vi "Autonomous Independent.vi"() -> ()   [LabVIEW 2017]
doc: "This VI is called when autonomous begins, and will automatically be terminated when autonomous ends. You can carry out timed or sensor driven robot movement independently without needing to return to the caller."
uses:
  Public/Documents/Cross The Road Electronics/Phoenix-LabVIEW/Motor Controller/Controls/CTRE_Phoenix_MotorControl_ControlMode.ctl
  <vilib>/Rock Robotics/WPI/Solenoid/WPI_SolenoidValue.ctl
  <vilib>/Rock Robotics/WPI/Utilities/WPI_GetSetVariantRefNum.vi
  <vilib>/Rock Robotics/Network Tables/NT Read String.vi
  <vilib>/Rock Robotics/Network Tables/NT Write Numeric Array.vi
  <vilib>/Rock Robotics/WPI/RobotDrive/WPI_RobotDriveArcadeDrive_Standard(NoSaturation).vi
  <vilib>/addons/control/pid/pid.llb/PID (DBL).vi
  <vilib>/Rock Robotics/WPI/Solenoid/WPI_SolenoidSetEnum.vi
  <vilib>/addons/control/pid/NI_PID_pid.lvlib
  <vilib>/Rock Robotics/WPI/ThirdParty/Sensors/ADIS16448 IMU/ADIS16448_IMU.lvlib
panel:
  out "Current Movement, for debugging":T1 {"Y Joystick Value" scale=1.0..-1.0; "X Joystick Value" scale=-1.0..1.0}
  in  "Array of robot movements":T2(array[cluster])=[{"X Joystick Value"=0.39393939393939403, "Y Joystick Value"=0.0, "Delay (sec)"=1.0, "Movement Name"="turn"}, {"X Joystick Value"=-0.3737373737373737, "Y Joystick Value"=0.0, "Delay (sec)"=1.0, "Movement Name"="turn back"}] {"Y Joystick Value" scale=1.0..-1.0; "X Joystick Value" scale=-1.0..1.0}
  # "Be sure to right-click and choose Data Operations>>Make Current Value default if you want to save the array values with the VI"
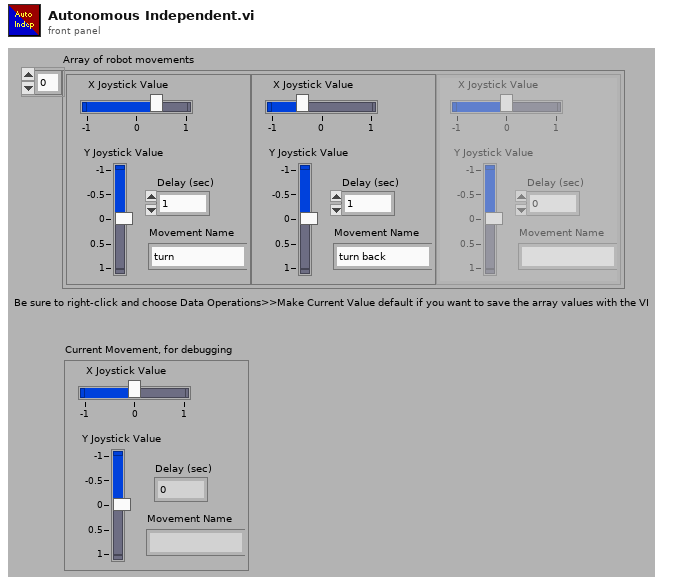
[diagram p1: front panel]
types:
  T1 = cluster{"X Joystick Value":dbl, "Y Joystick Value":dbl, "Delay (sec)":dbl, "Movement Name":string}
  T2 = cluster{"X Joystick Value":dbl, "Y Joystick Value":dbl, "Delay (sec)":dbl, "Movement Name":string}[]
  T3 = typedef "WPI_JoystickDevRef.ctl" = cluster{"Device":T4}
  T4 = typedef "WPI_JoystickDeviceEnum.ctl" = enum16{"USB 0", "USB 1", "USB 2", "USB 3", "USB 4", "USB 5"}
  T5 = typedef "ADIS16448_IMU.lvlib/ADI_IMU_ADIS16448_IMUDevRef.ctl" = cluster{"DevStatus":errorcluster, "Handle":i32, "SPI Bus":T6, "Device Found":bool, "Device Ready":bool, "Yaw Axis":enum16{"X", "Y", "Z"}, "AHRS Algorithm":enum16{"Complementary", "Madgwick"}, "Serial":u16, "Lot ID 2":u16, "Lot ID 1":u16, "Bytes Per Sample":u16, "Calibrate On Open?":bool}
  T6 = typedef "spi_bus.ctl" = enum16{"SPI On-Board, CS0", "SPI On-Board, CS1", "SPI On-Board, CS2", "SPI On-Board, CS3", "SPI MXP", "Invalid"}
  T7 = typedef "WPI_RobotDriveDevRef.ctl" = cluster{"DevStatus":errorcluster, "Motors[]":T8[], "Square Inputs":bool, "Max Output":dbl}
  T8 = typedef "WPI_MotorControlDeviceRef.ctl" = cluster{"DeviceStatus":errorcluster, "Type":T9, "PWM":cluster{"PWM Channel":T10, "DeadBand":T11}, "CAN":cluster{"Device Number":u8, "SetOutput VI Ref":variant, "GetOutput VI Ref":variant, "Enable VI Ref":variant, "Disable VI Ref":variant, "Data":variant}, "Invert":bool, "DIO PWM":cluster{"PWM \"Enable\" Channel":T10, "DIOChannel":T12, "PWM Rate":dbl}}
  T9 = typedef "WPI_MotorControlType.ctl" = enum16{"PWM", "CAN", "DIO PWM"}
  T10 = typedef "FPGA_DIOPWMChannel.ctl" = enum8{"PWM 0", "PWM 1", "PWM 2", "PWM 3", "PWM 4", "PWM 5", "PWM 6", "PWM 7", "PWM 8", "PWM 9", "PWM MXP 0", "PWM MXP 1", "PWM MXP 2", "PWM MXP 3", "PWM MXP 4", "PWM MXP 5", "PWM MXP 6", "PWM MXP 7", "PWM MXP 8", "PWM MXP 9", "Invalid"}
  T11 = typedef "WPI_PWMDeadband.ctl" = cluster{"Name":string, "maxPositivePwm":i32, "minPositivePwm":i32, "centerPwm":i32, "maxNegativePwm":i32, "minNegativePwm":i32, "angularRange":u16}
  T12 = typedef "FPGA_DIOChannel.ctl" = enum8{"DIO 0", "DIO 1", "DIO 2", "DIO 3", "DIO 4", "DIO 5", "DIO 6", "DIO 7", "DIO 8", "DIO 9", "DIO MXP 0", "DIO MXP 1", "DIO MXP 2", "DIO MXP 3", "DIO MXP 4", "DIO MXP 5", "DIO MXP 6", "DIO MXP 7", "DIO MXP 8", "DIO MXP 9", "DIO MXP 10", "DIO MXP 11", "DIO MXP 12", "DIO MXP 13", "DIO MXP 14", "DIO MXP 15", "SPI Port CS1", "SPI Port CS2", "SPI Port CS3", "SPI Port MISO", "SPI Port MOSI", "Invalid"}
  T13 = typedef "WPI_SolenoidDevRef.ctl" = cluster{"DevStatus":errorcluster, "Pneumatics Control Module":u8, "Forward Solenoid Channel":T14, "Reverse Solenoid Channel":T14}
  T14 = typedef "WPI_SolenoidChannel.ctl" = enum8{"Solenoid 0", "Solenoid 1", "Solenoid 2", "Solenoid 3", "Solenoid 4", "Solenoid 5", "Solenoid 6", "Solenoid 7", "Invalid"}
  T15 = cluster{"proportional gain (Kc)":dbl, "integral time (Ti, min)":dbl, "derivative time (Td, min)":dbl}
  T16 = typedef "WPI_SolenoidValue.ctl" = enum16{"Off", "On", "Forward", "Reverse"}
  T17 = cluster{"X Angle":dbl, "Y Angle":dbl, "Z Angle":dbl}
  T18 = typedef "CTRE_Phoenix_MotorControl_ControlMode.ctl" = u16
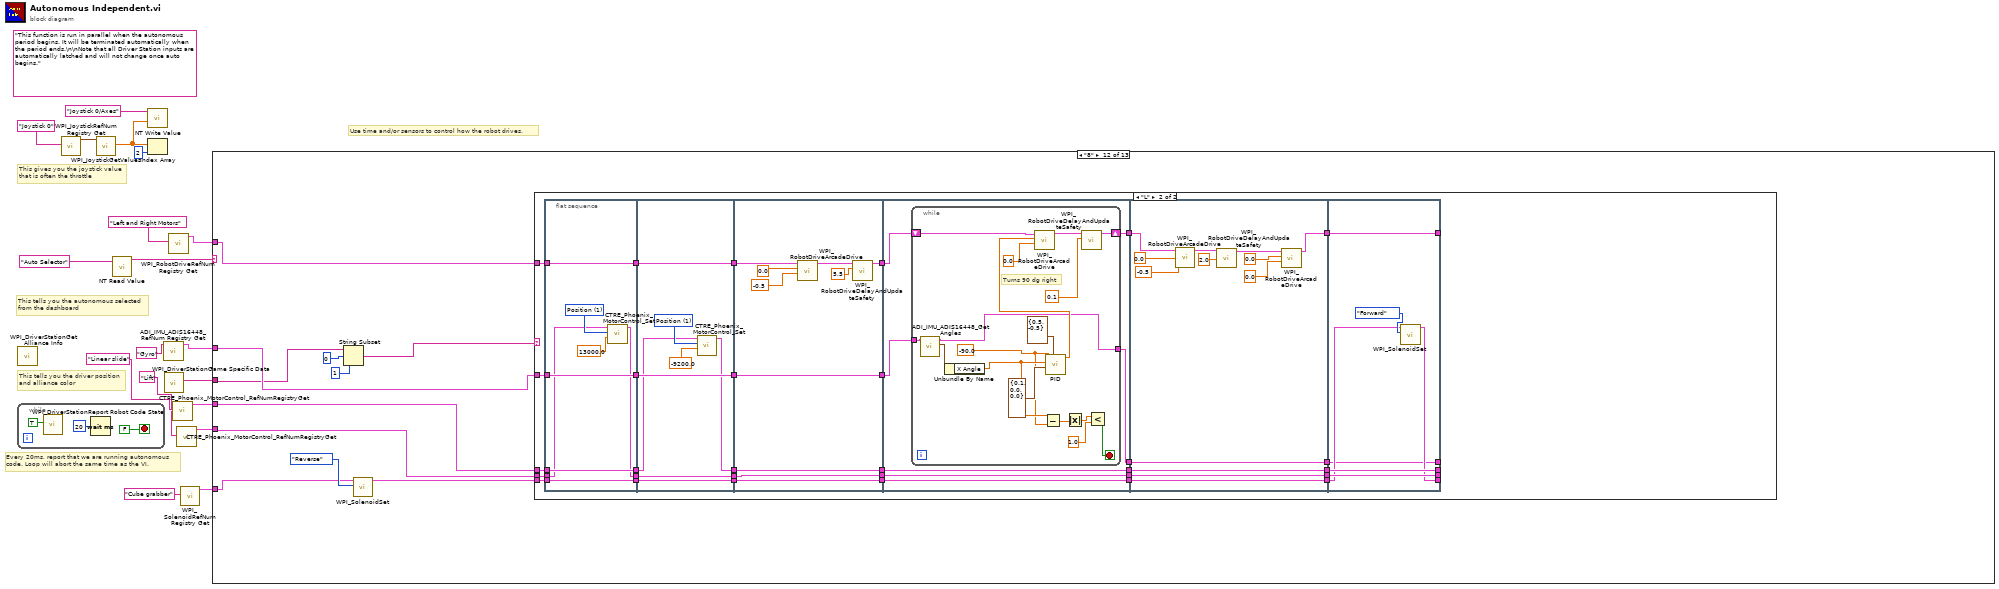
[diagram p0: block diagram]
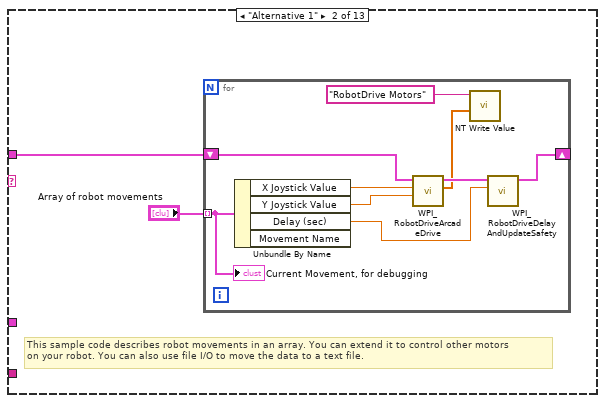
[diagram p3: hidden frame]
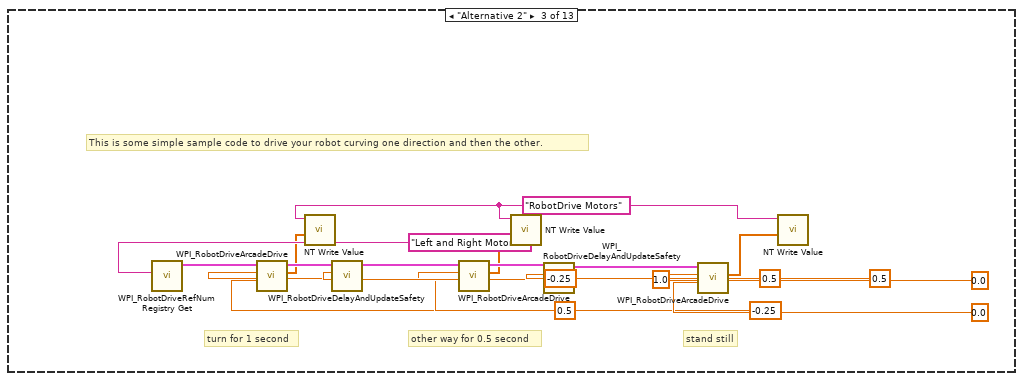
[diagram p4: hidden frame]
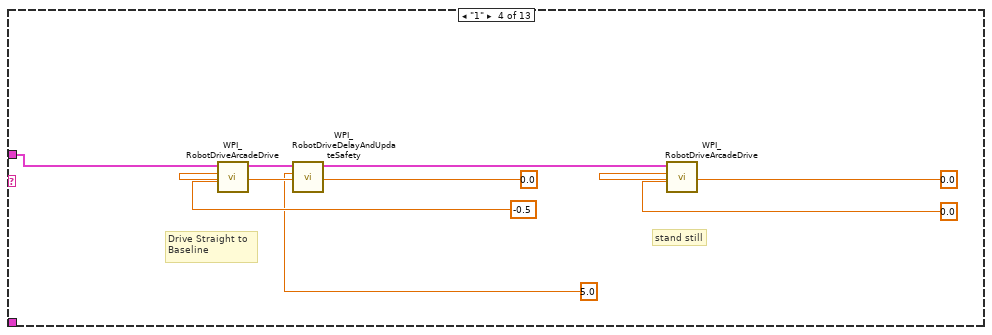
[diagram p5: hidden frame]
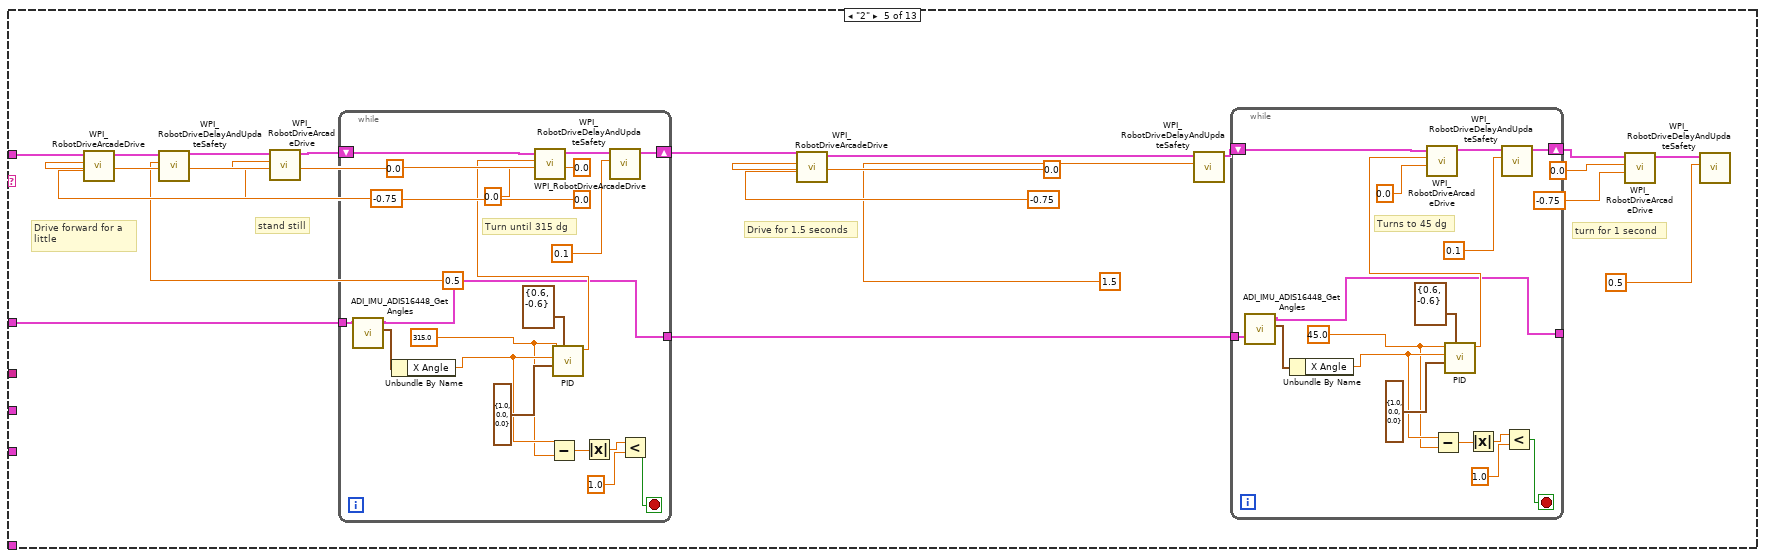
[diagram p6: hidden frame]
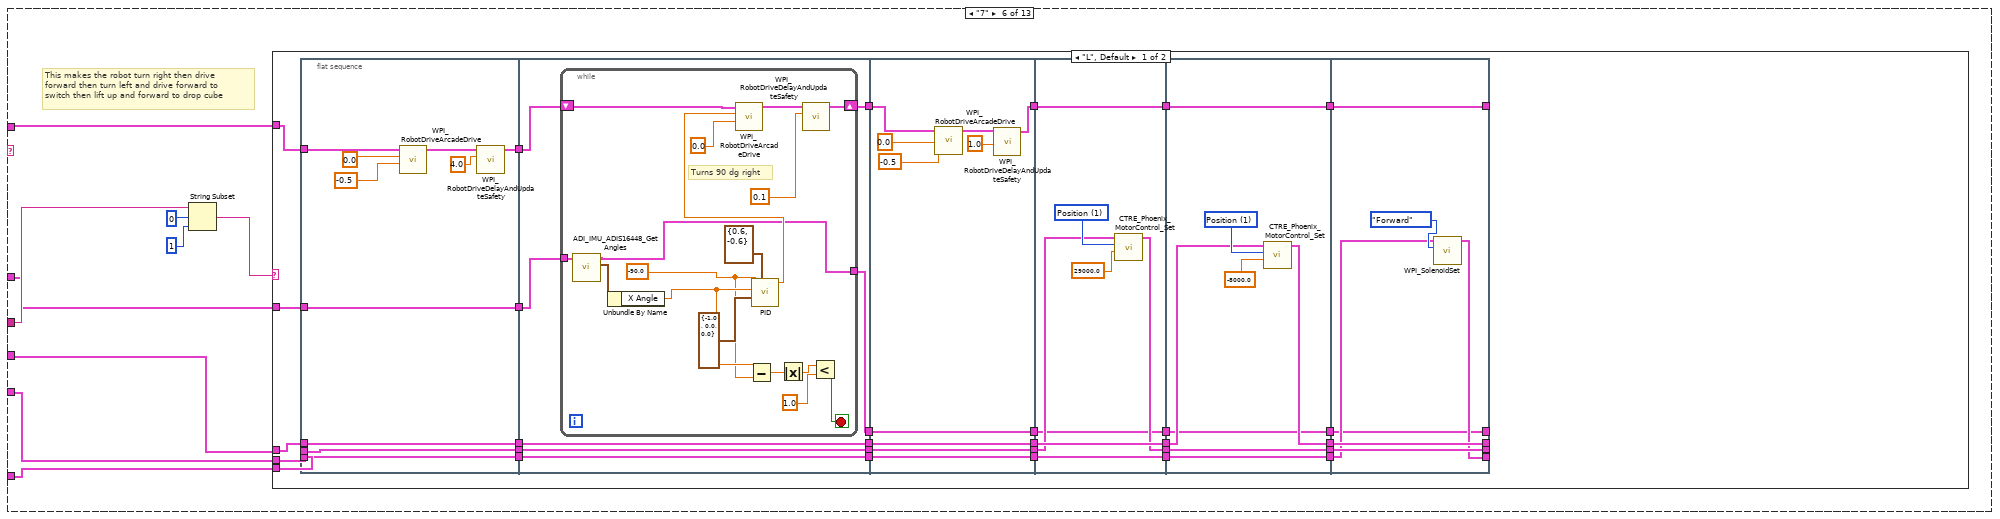
[diagram p7: hidden frame]
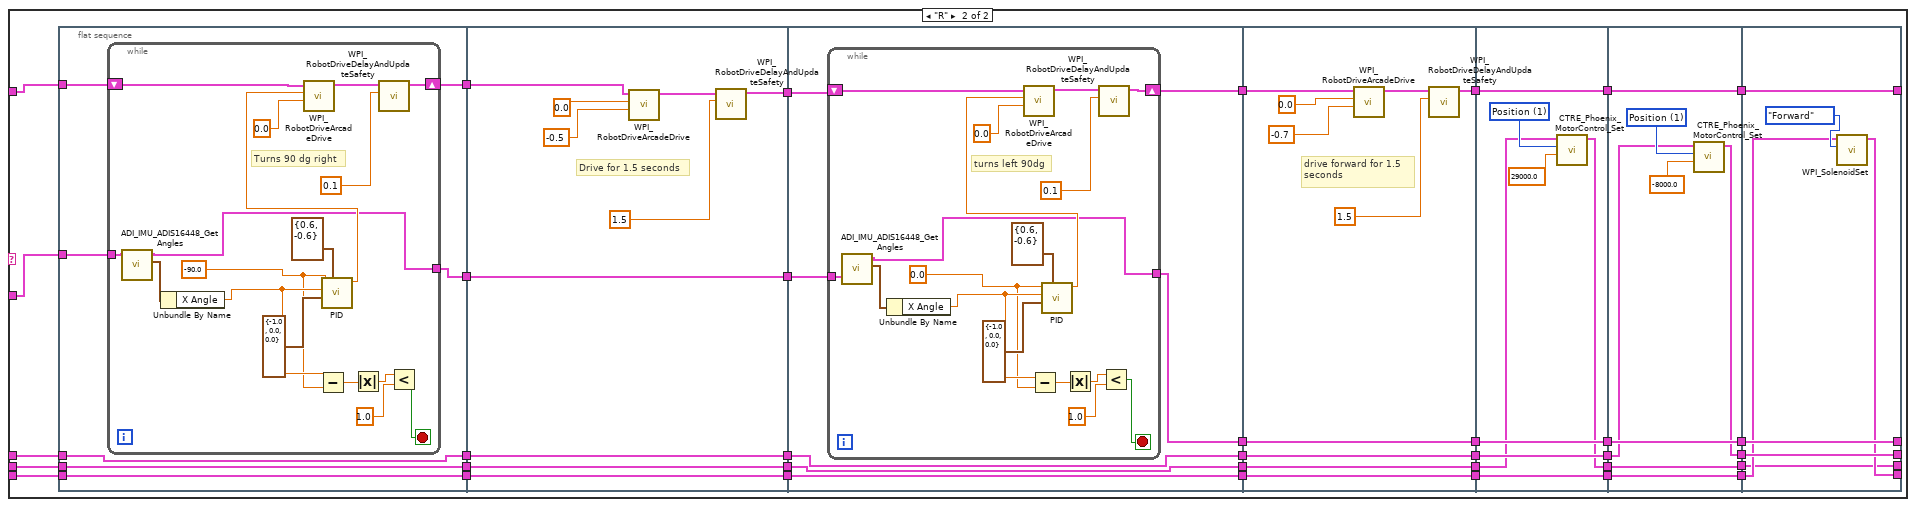
[diagram p8: hidden frame]
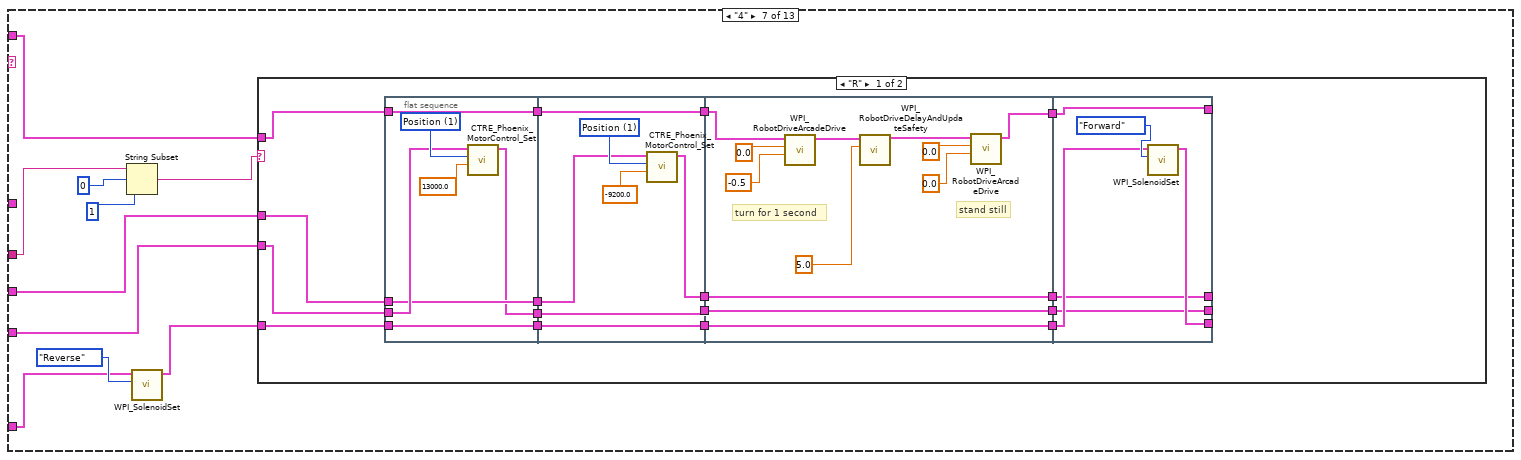
[diagram p9: hidden frame]
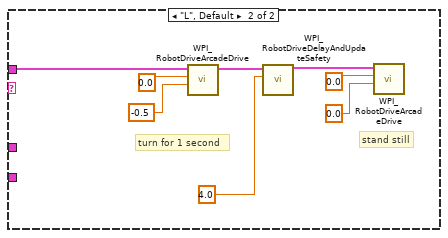
[diagram p10: hidden frame]
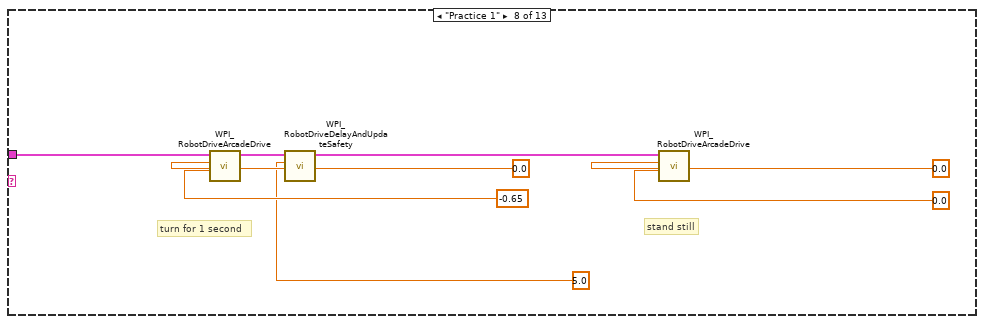
[diagram p11: hidden frame]
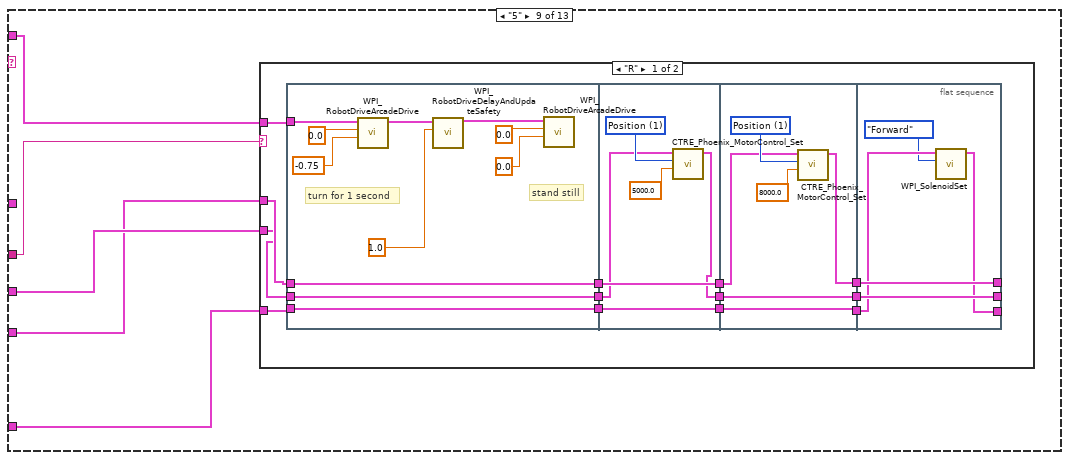
[diagram p12: hidden frame]
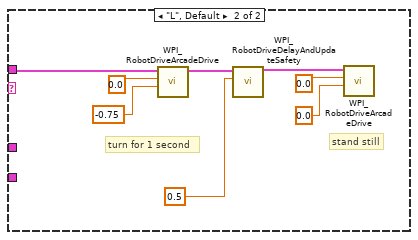
[diagram p13: hidden frame]
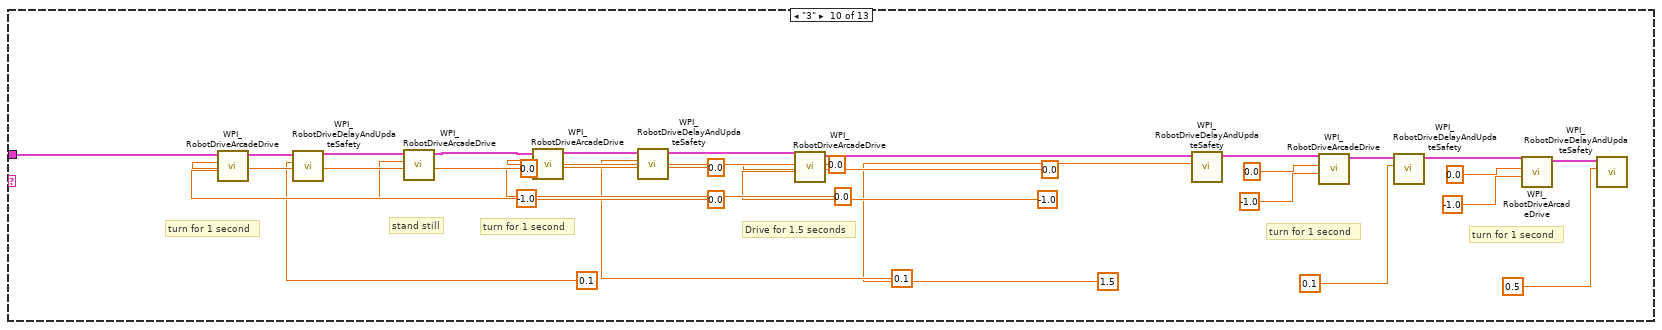
[diagram p14: hidden frame]
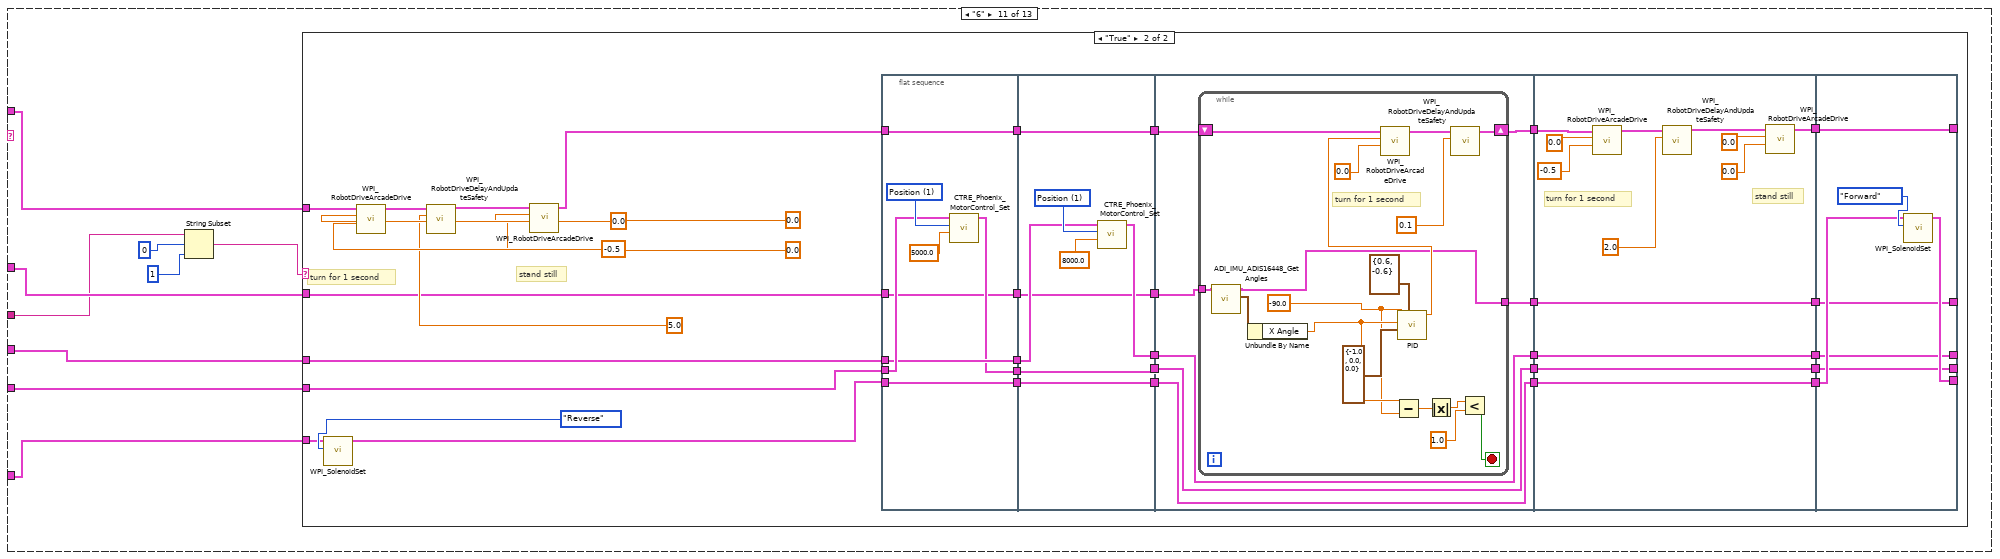
[diagram p15: hidden frame]
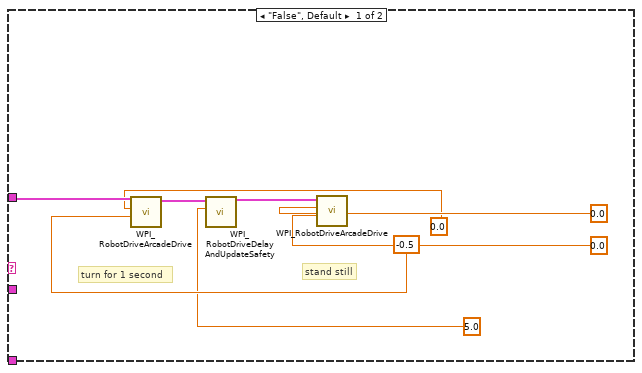
[diagram p16: hidden frame]
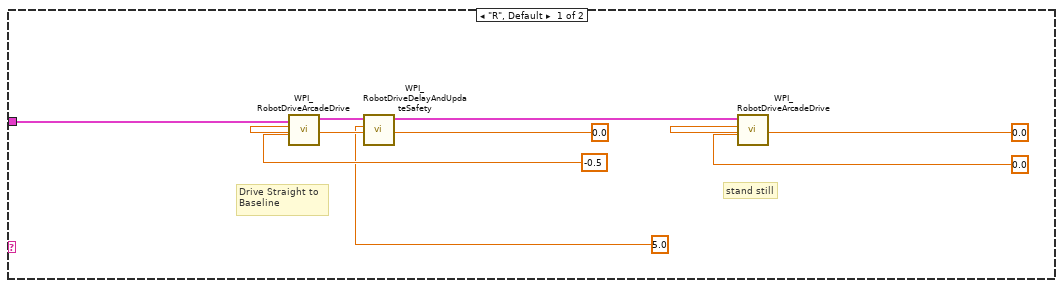
[diagram p17: hidden frame]
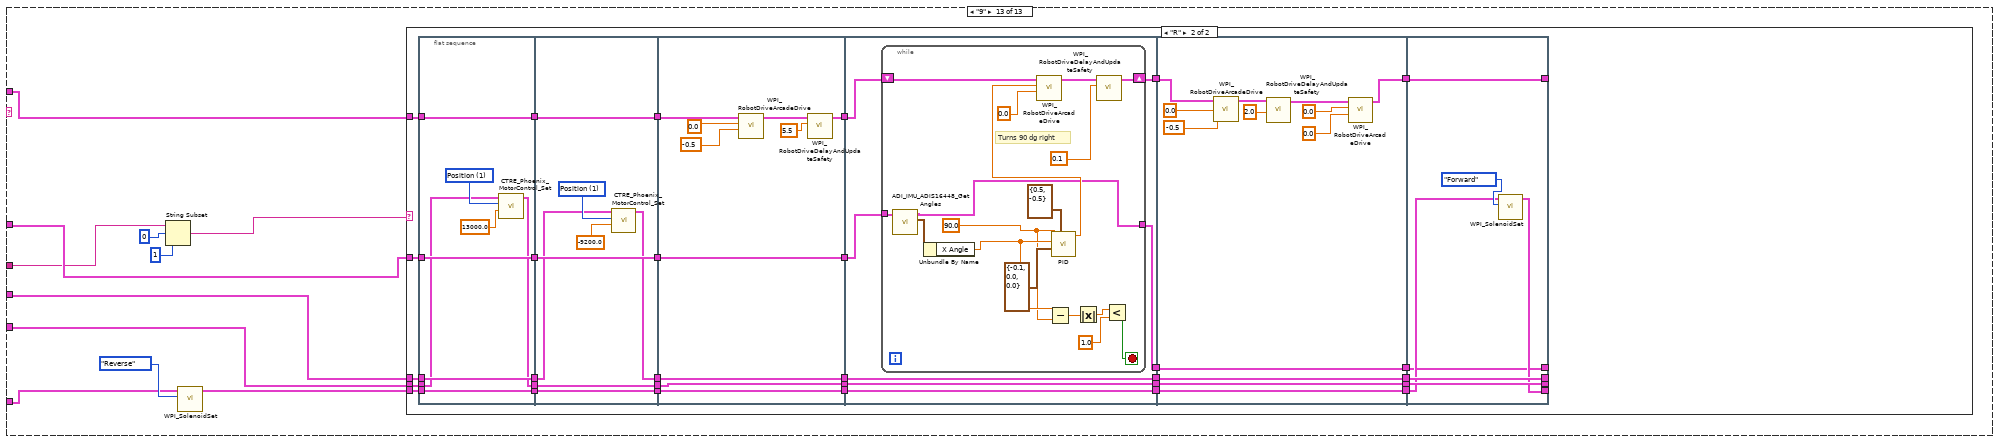
[diagram p18: hidden frame]
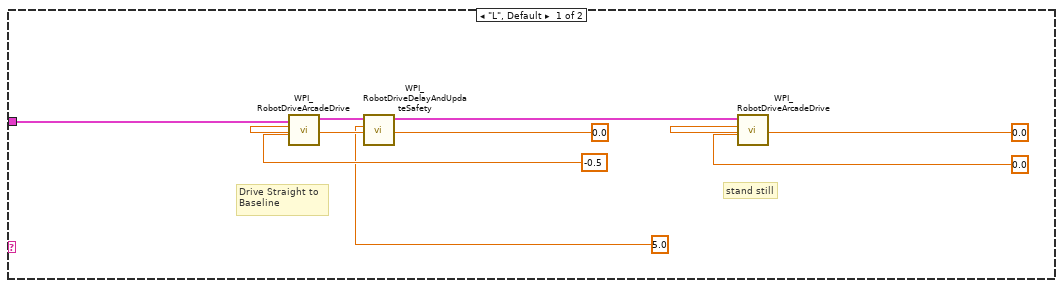
[diagram p19: hidden frame]
diagram:
  (unwired) "This function is run in parallel when the autonomous period begins. It will be terminated automatically when the period ends.\n\nNote that all Driver Station inputs are automatically latched and will not change once auto begins."
  # "This tells you the autonomous selected\nfrom the dashboard"
  # "Every 20ms, report that we are running autonomous\ncode. Loop will abort the same time as the VI."
  # "This gives you the joystick value\nthat is often the throttle"
  # "Use time and/or sensors to control how the robot drives."
  # "This tells you the driver position\nand alliance color"
  n1 = while {
    stop <- FALSE stop-if-true
    n2 = call <vilib>:"WPI_DriverStationReport Robot Code State.vi"("Autonomous"=TRUE) -> ()  [unwired: 10 in, 1 out]
    n3 = Wait (ms)(milliseconds to wait=u32 20) -> ()  [unwired: 1 out]
  }
  n4 = call <vilib>:"WPI_DriverStationGet Alliance Info.vi"() -> ()  [unwired: 12 out]
  n5 = call <vilib>:"WPI_JoystickRefNum Registry Get.vi"("refnum name"="Joystick 0") -> ("JoystickDevRef"=w17:T3)  [unwired: 1 in, 9 out]
  n6 = call <vilib>:"WPI_JoystickGetValues.vi"("JoystickDevRef"=w17) -> ("Axes"=w13:dbl[])  [unwired: 6 in, 4 out]
  n7 = call-poly <vilib>:"NT Read Value.vi"("Name"="Auto Selector") -> ("String"=w14:string)  [unwired: 9 in, 1 out]
  n8 = call-poly <vilib>:"NT Write Value.vi"("Numeric Array"=w13, "Name"="Joystick 0/Axes") -> ()  [unwired: 9 in, 1 out]
  n9 = Index Array(array=w13, index=2) -> ()  [unwired: 1 out]
  n10 = call <vilib>:"ADI_IMU_ADIS16448_RefNum Registry Get.vi"("refnum name"="Gyro") -> ("ADI IMU DevRef"=w8:T5)  [unwired: 9 in, 1 out]
  n11 = call <vilib>:"WPI_DriverStationGame Specific Data.vi"() -> ("Game Specific Data"=w7:string)  [unwired: 11 in]
  n12 = call <vilib>:"WPI_RobotDriveRefNum Registry Get.vi"("refnum name"="Left and Right Motors") -> ("RobotDriveDevRef"=w10:T7)  [unwired: 1 in, 9 out]
  n13 = call "CTRE_Phoenix_MotorControl_RefNumRegistryGet.vi"("refnum name"="Linear slide") -> ("PhoenixMotorControlDevRef"=w5:T8)  [unwired: 9 in, 1 out]
  n14 = call "CTRE_Phoenix_MotorControl_RefNumRegistryGet.vi"("refnum name"="Lift") -> ("PhoenixMotorControlDevRef"=w4:T8)  [unwired: 9 in, 1 out]
  n15 = call <vilib>:"WPI_SolenoidRefNum Registry Get.vi"("refnum name"="Cube grabber") -> ("SolenoidDevRef"=w1:T13)  [unwired: 9 in, 1 out]
  n16 = case shown="\"8\"" w14 {
    tunnel: w10 -> [_ w22 _ w51 w72 w123 w352 w413 w425 w475 w511 w617 w741]
    tunnel: w8 -> [_ _ _ _ w63 w119 _ _ _ _ w508 w620 w742]
    tunnel: w7 -> [_ _ _ _ _ w120 w356 _ w424 _ w504 w615 w740]
    tunnel: w5 -> [_ _ _ _ _ w117 w350 _ w422 _ w509 w619 w744]
    tunnel: w4 -> [_ _ _ _ _ w116 w351 _ w421 _ w510 w618 w743]
    tunnel: w1 -> [_ _ _ _ _ w115 w348 _ w423 _ w507 w616 w735]
    frame "Do nothing", Default {
    }
    frame "Alternative 1" {
      # "This sample code describes robot movements in an array. You can extend it to control other motors\non your robot. You can also use file I/O to move the data to a text file."
      n17 = for {
        shift-right: [w30] -> _
        shift-left: w22 -> [w31]
        tunnel: "Array of robot movements" -> [w26] mode=indexing
        n18 = Unbundle By Name(w26) -> ("X Joystick Value"=w29:dbl, "Y Joystick Value"=w28:dbl, "Delay (sec)"=w27:dbl)  [unwired: 1 out]
        n19 = call-poly <vilib>:"WPI_RobotDriveArcadeDrive.vi"("Y axis value"=w28, "X axis value"=w29, "RobotDriveDevRef"=w31) -> ("Motor Values"=w24:dbl[], "RobotDriveDevRef"=w32:T7)  [unwired: 1 in, 6 out]
        n20 = call-poly <vilib>:"NT Write Value.vi"("Numeric Array"=w24, "Name"="RobotDrive Motors") -> ()  [unwired: 9 in, 1 out]
        n21 = call <vilib>:"WPI_RobotDriveDelayAndUpdateSafety.vi"("Delay (s)"=w27, "RobotDriveDevRef"=w32) -> ("RobotDriveDevRef 2"=w30:T7)  [unwired: 8 in, 1 out]
        "Current Movement, for debugging" <- w26
      }
    }
    frame "Alternative 2" {
      w34 = "RobotDrive Motors" ("Name")
      # "This is some simple sample code to drive your robot curving one direction and then the other."
      # "stand still"
      # "other way for 0.5 second"
      # "turn for 1 second"
      n22 = call <vilib>:"WPI_RobotDriveRefNum Registry Get.vi"("refnum name"="Left and Right Motors") -> ("RobotDriveDevRef"=w50:T7)  [unwired: 1 in, 9 out]
      n23 = call-poly <vilib>:"WPI_RobotDriveArcadeDrive.vi"("Y axis value"=0.5 ("X axis value"), "X axis value"=-0.25, "RobotDriveDevRef"=w50) -> ("Motor Values"=w33:dbl[], "RobotDriveDevRef"=w43:T7)  [unwired: 1 in, 6 out]
      n24 = call-poly <vilib>:"NT Write Value.vi"("Numeric Array"=w33, "Name"=w34) -> ()  [unwired: 9 in, 1 out]
      n25 = call <vilib>:"WPI_RobotDriveDelayAndUpdateSafety.vi"("Delay (s)"=1.0, "RobotDriveDevRef"=w43) -> ("RobotDriveDevRef 2"=w44:T7)  [unwired: 8 in, 1 out]
      n26 = call-poly <vilib>:"WPI_RobotDriveArcadeDrive.vi"("Y axis value"=-0.25 ("X axis value"), "X axis value"=0.5, "RobotDriveDevRef"=w44) -> ("Motor Values"=w35:dbl[], "RobotDriveDevRef"=w45:T7)  [unwired: 1 in, 6 out]
      n27 = call-poly <vilib>:"NT Write Value.vi"("Numeric Array"=w35, "Name"=w34) -> ()  [unwired: 9 in, 1 out]
      n28 = call <vilib>:"WPI_RobotDriveDelayAndUpdateSafety.vi"("Delay (s)"=0.5, "RobotDriveDevRef"=w45) -> ("RobotDriveDevRef 2"=w46:T7)  [unwired: 8 in, 1 out]
      n29 = call-poly <vilib>:"WPI_RobotDriveArcadeDrive.vi"("Y axis value"=0.0 ("X axis value"), "X axis value"=0.0, "RobotDriveDevRef"=w46) -> ("Motor Values"=w36:dbl[])  [unwired: 1 in, 7 out]
      n30 = call-poly <vilib>:"NT Write Value.vi"("Numeric Array"=w36, "Name"=w34) -> ()  [unwired: 9 in, 1 out]
    }
    frame "1" {
      # "stand still"
      # "Drive Straight to \nBaseline"
      n31 = call-poly <vilib>:"WPI_RobotDriveArcadeDrive.vi"("Y axis value"=-0.5 ("X axis value"), "X axis value"=0.0, "RobotDriveDevRef"=w51) -> ("RobotDriveDevRef"=w54:T7)  [unwired: 1 in, 7 out]
      n32 = call <vilib>:"WPI_RobotDriveDelayAndUpdateSafety.vi"("Delay (s)"=5.0, "RobotDriveDevRef"=w54) -> ("RobotDriveDevRef 2"=w52:T7)  [unwired: 8 in, 1 out]
      n33 = call-poly <vilib>:"WPI_RobotDriveArcadeDrive.vi"("Y axis value"=0.0 ("X axis value"), "X axis value"=0.0, "RobotDriveDevRef"=w52) -> ()  [unwired: 1 in, 8 out]
    }
    frame "2" {
      # "turn for 1 second"
      # "Drive for 1.5 seconds"
      # "stand still"
      # "Drive forward for a \nlittle"
      n34 = call-poly <vilib>:"WPI_RobotDriveArcadeDrive.vi"("Y axis value"=-0.75 ("X axis value"), "X axis value"=0.0, "RobotDriveDevRef"=w72) -> ("RobotDriveDevRef"=w76:T7)  [unwired: 1 in, 7 out]
      n35 = call <vilib>:"WPI_RobotDriveDelayAndUpdateSafety.vi"("Delay (s)"=0.5, "RobotDriveDevRef"=w76) -> ("RobotDriveDevRef 2"=w74:T7)  [unwired: 8 in, 1 out]
      n36 = call-poly <vilib>:"WPI_RobotDriveArcadeDrive.vi"("Y axis value"=0.0 ("X axis value"), "X axis value"=0.0, "RobotDriveDevRef"=w74) -> ("RobotDriveDevRef"=w73:T7)  [unwired: 1 in, 7 out]
      n37 = while {
        tunnel: w63 -> [w106]
        shift-right: [w110] -> w68
        shift-left: w73 -> [w111]
        tunnel: [w105] -> w60
        stop <- w99 stop-if-true
        w102 = 315.0 ("setpoint")
        # "Turn until 315 dg"
        n38 = call <vilib>:"ADI_IMU_ADIS16448_Get Angles.vi"("ADI IMU DevRef"=w106) -> ("IMU Angles Out"=w104:T17, "ADI IMU DevRef Out"=w105:T5)  [unwired: 7 in, 2 out]
        n39 = Unbundle By Name(w104) -> ("X Angle"=w103:dbl)
        n40 = Subtract(x=w103, y=w102) -> (x-y=w101:dbl)
        n41 = call-poly <vilib>:"PID.vi"("output range"=cluster{"output high":dbl, "output low":dbl} {"output high"=0.6, "output low"=-0.6}, "PID gains"=T15 {"proportional gain (Kc)"=1.0, "integral time (Ti, min)"=0.0, "derivative time (Td, min)"=0.0}, "process variable"=w103, "setpoint"=w102) -> ("output"=w107:dbl)  [unwired: 6 in, 1 out]
        n42 = call-poly <vilib>:"WPI_RobotDriveArcadeDrive.vi"("Y axis value"=0.0 ("X axis value"), "X axis value"=w107, "RobotDriveDevRef"=w111) -> ("RobotDriveDevRef"=w113:T7)  [unwired: 1 in, 7 out]
        n43 = Absolute Value(x=w101) -> (abs(x)=w100:dbl)
        n44 = call <vilib>:"WPI_RobotDriveDelayAndUpdateSafety.vi"("Delay (s)"=0.1, "RobotDriveDevRef"=w113) -> ("RobotDriveDevRef 2"=w110:T7)  [unwired: 8 in, 1 out]
        n45 = Less?(x=w100, y=1.0) -> (x < y?=w99:bool)
      }
      n46 = call-poly <vilib>:"WPI_RobotDriveArcadeDrive.vi"("Y axis value"=-0.75 ("X axis value"), "X axis value"=0.0, "RobotDriveDevRef"=w68) -> ("RobotDriveDevRef"=w69:T7)  [unwired: 1 in, 7 out]
      n47 = call <vilib>:"WPI_RobotDriveDelayAndUpdateSafety.vi"("Delay (s)"=1.5, "RobotDriveDevRef"=w69) -> ("RobotDriveDevRef 2"=w62:T7)  [unwired: 8 in, 1 out]
      n48 = while {
        shift-right: [w93] -> w61
        shift-left: w62 -> [w94]
        tunnel: [w88] -> _
        tunnel: w60 -> [w89]
        stop <- w81 stop-if-true
        w82 = 45.0 ("setpoint")
        # "Turns to 45 dg"
        n49 = call <vilib>:"ADI_IMU_ADIS16448_Get Angles.vi"("ADI IMU DevRef"=w89) -> ("IMU Angles Out"=w87:T17, "ADI IMU DevRef Out"=w88:T5)  [unwired: 7 in, 2 out]
        n50 = Unbundle By Name(w87) -> ("X Angle"=w83:dbl)
        n51 = Subtract(x=w83, y=w82) -> (x-y=w86:dbl)
        n52 = call-poly <vilib>:"PID.vi"("output range"=cluster{"output high":dbl, "output low":dbl} {"output high"=0.6, "output low"=-0.6}, "PID gains"=T15 {"proportional gain (Kc)"=1.0, "integral time (Ti, min)"=0.0, "derivative time (Td, min)"=0.0}, "process variable"=w83, "setpoint"=w82) -> ("output"=w90:dbl)  [unwired: 6 in, 1 out]
        n53 = call-poly <vilib>:"WPI_RobotDriveArcadeDrive.vi"("Y axis value"=0.0 ("X axis value"), "X axis value"=w90, "RobotDriveDevRef"=w94) -> ("RobotDriveDevRef"=w96:T7)  [unwired: 1 in, 7 out]
        n54 = Absolute Value(x=w86) -> (abs(x)=w85:dbl)
        n55 = call <vilib>:"WPI_RobotDriveDelayAndUpdateSafety.vi"("Delay (s)"=0.1, "RobotDriveDevRef"=w96) -> ("RobotDriveDevRef 2"=w93:T7)  [unwired: 8 in, 1 out]
        n56 = Less?(x=w85, y=1.0) -> (x < y?=w81:bool)
      }
      n57 = call-poly <vilib>:"WPI_RobotDriveArcadeDrive.vi"("Y axis value"=-0.75 ("X axis value"), "X axis value"=0.0, "RobotDriveDevRef"=w61) -> ("RobotDriveDevRef"=w65:T7)  [unwired: 2 in, 6 out]
      n58 = call <vilib>:"WPI_RobotDriveDelayAndUpdateSafety.vi"("Delay (s)"=0.5, "RobotDriveDevRef"=w65) -> ()  [unwired: 8 in, 2 out]
    }
    frame "7" {
      # "This makes the robot turn right then drive \nforward then turn left and drive forward to \nswitch then lift up and forward to drop cube"
      n59 = String Subset(string=w120, offset (0)=0, length (rest)=1 ("length (rest)")) -> (substring=w118:string)
      n60 = case shown="\"L\", Default" w118 {
        tunnel: w123 -> [w153 w254]
        tunnel: w119 -> [w152 w253]
        tunnel: w117 -> [w145 w241]
        tunnel: w116 -> [w147 w236]
        tunnel: w115 -> [w149 w231]
        frame "L", Default {
          n61 = flat-sequence {
            tunnel: w153 -> [w163]
            tunnel: [w161] -> w151
            tunnel: [w157] -> w150
            tunnel: w152 -> [w157]
            tunnel: w149 -> [w156]
            tunnel: [w156] -> w148
            tunnel: w147 -> [w155]
            tunnel: [w155] -> w146
            tunnel: w145 -> [w154]
            tunnel: [w154] -> w144
            tunnel: w151 -> [w167]
            tunnel: w150 -> [w166]
            tunnel: w148 -> [w170]
            tunnel: [w170] -> w133
            tunnel: w146 -> [w169]
            tunnel: [w169] -> w131
            tunnel: w144 -> [w168]
            tunnel: [w168] -> w129
            tunnel: [w165] -> w127
            tunnel: [w164] -> w125
            tunnel: w133 -> [w197]
            tunnel: [w197] -> w132
            tunnel: w131 -> [w196]
            tunnel: [w196] -> w130
            tunnel: w129 -> [w195]
            tunnel: [w195] -> w128
            tunnel: w127 -> [w192]
            tunnel: [w191] -> w126
            tunnel: w125 -> [w194]
            tunnel: [w194] -> w124
            tunnel: w132 -> [w205]
            tunnel: [w205] -> w143
            tunnel: w130 -> [w201]
            tunnel: [w200] -> w141
            tunnel: w128 -> [w204]
            tunnel: [w204] -> w139
            tunnel: w126 -> [w199]
            tunnel: [w199] -> w136
            tunnel: [w198] -> w134
            tunnel: w124 -> [w198]
            tunnel: w143 -> [w213]
            tunnel: [w213] -> w142
            tunnel: w141 -> [w212]
            tunnel: [w212] -> w140
            tunnel: w139 -> [w209]
            tunnel: [w208] -> w138
            tunnel: [w207] -> w137
            tunnel: w136 -> [w207]
            tunnel: [w206] -> w135
            tunnel: w134 -> [w206]
            tunnel: w142 -> [w217]
            tunnel: w140 -> [w220]
            tunnel: [w220] -> _
            tunnel: w138 -> [w219]
            tunnel: [w219] -> _
            tunnel: [w216] -> _
            tunnel: [w215] -> _
            tunnel: w137 -> [w215]
            tunnel: [w214] -> _
            tunnel: w135 -> [w214]
            frame #0 {
              n62 = call-poly <vilib>:"WPI_RobotDriveArcadeDrive.vi"("Y axis value"=-0.5, "X axis value"=0.0, "RobotDriveDevRef"=w163) -> ("RobotDriveDevRef"=w162:T7)  [unwired: 6 in, 2 out]
              n63 = call <vilib>:"WPI_RobotDriveDelayAndUpdateSafety.vi"("Delay (s)"=4.0, "RobotDriveDevRef"=w162) -> ("RobotDriveDevRef 2"=w161:T7)  [unwired: 8 in, 1 out]
            }
            frame #1 {
              n64 = while {
                tunnel: w166 -> [w179]
                shift-right: [w183] -> w165
                shift-left: w167 -> [w184]
                tunnel: [w178] -> w164
                stop <- w172 stop-if-true
                w175 = -90.0 ("setpoint")
                # "Turns 90 dg right"
                n65 = call <vilib>:"ADI_IMU_ADIS16448_Get Angles.vi"("ADI IMU DevRef"=w179) -> ("IMU Angles Out"=w177:T17, "ADI IMU DevRef Out"=w178:T5)  [unwired: 7 in, 2 out]
                n66 = Unbundle By Name(w177) -> ("X Angle"=w176:dbl)
                n67 = Subtract(x=w176, y=w175) -> (x-y=w174:dbl)
                n68 = call-poly <vilib>:"PID.vi"("output range"=cluster{"output high":dbl, "output low":dbl} {"output high"=0.6, "output low"=-0.6}, "PID gains"=T15 {"proportional gain (Kc)"=-1.0, "integral time (Ti, min)"=0.0, "derivative time (Td, min)"=0.0}, "process variable"=w176, "setpoint"=w175) -> ("output"=w180:dbl)  [unwired: 6 in, 1 out]
                n69 = call-poly <vilib>:"WPI_RobotDriveArcadeDrive.vi"("Y axis value"=0.0 ("X axis value"), "X axis value"=w180, "RobotDriveDevRef"=w184) -> ("RobotDriveDevRef"=w186:T7)  [unwired: 1 in, 7 out]
                n70 = Absolute Value(x=w174) -> (abs(x)=w173:dbl)
                n71 = call <vilib>:"WPI_RobotDriveDelayAndUpdateSafety.vi"("Delay (s)"=0.1, "RobotDriveDevRef"=w186) -> ("RobotDriveDevRef 2"=w183:T7)  [unwired: 8 in, 1 out]
                n72 = Less?(x=w173, y=1.0) -> (x < y?=w172:bool)
              }
            }
            frame #2 {
              n73 = call-poly <vilib>:"WPI_RobotDriveArcadeDrive.vi"("Y axis value"=-0.5, "X axis value"=0.0, "RobotDriveDevRef"=w192) -> ("RobotDriveDevRef"=w193:T7)  [unwired: 6 in, 2 out]
              n74 = call <vilib>:"WPI_RobotDriveDelayAndUpdateSafety.vi"("Delay (s)"=1.0, "RobotDriveDevRef"=w193) -> ("RobotDriveDevRef 2"=w191:T7)  [unwired: 8 in, 1 out]
            }
            frame #3 {
              w202 = T18 1 items=["PercentOutput"=0, "Position"=1, "Velocity"=2, "Current"=3, "Follower"=5, "MotionProfile"=6, "MotionMagic"=7, "MotionMagicArc"=8, "MotionProfileArc"=10, "Disabled"=15] ("Control Mode")
              n75 = call "CTRE_Phoenix_MotorControl_Set.vi"("Output"=29000.0, "Control Mode"=w202, "PhoenixMotorControlDevRef"=w201) -> ("PhoenixMotorControlDevRef"=w200:T8)  [unwired: 7 in, 1 out]
            }
            frame #4 {
              w210 = T18 1 items=["PercentOutput"=0, "Position"=1, "Velocity"=2, "Current"=3, "Follower"=5, "MotionProfile"=6, "MotionMagic"=7, "MotionMagicArc"=8, "MotionProfileArc"=10, "Disabled"=15] ("Control Mode")
              n76 = call "CTRE_Phoenix_MotorControl_Set.vi"("Output"=-8000.0, "Control Mode"=w210, "PhoenixMotorControlDevRef"=w209) -> ("PhoenixMotorControlDevRef"=w208:T8)  [unwired: 7 in, 1 out]
            }
            frame #5 {
              n77 = call-poly <vilib>:"WPI_SolenoidSet.vi"("Value"=WPI_SolenoidValue."Forward", "SolenoidDevRef"=w217) -> ("SolenoidDevRef"=w216:T13)  [unwired: 8 in, 1 out]
            }
          }
        }
        frame "R" {
          n78 = flat-sequence {
            tunnel: [w262] -> w255
            tunnel: w254 -> [w261]
            tunnel: w253 -> [w260]
            tunnel: [w259] -> w251
            tunnel: w241 -> [w258]
            tunnel: [w258] -> w240
            tunnel: w236 -> [w257]
            tunnel: [w257] -> w235
            tunnel: w231 -> [w256]
            tunnel: [w256] -> w230
            tunnel: w255 -> [w284]
            tunnel: [w286] -> w252
            tunnel: w251 -> [w286]
            tunnel: [w283] -> w250
            tunnel: w240 -> [w282]
            tunnel: [w282] -> w239
            tunnel: w235 -> [w281]
            tunnel: [w281] -> w234
            tunnel: w230 -> [w280]
            tunnel: [w280] -> w229
            tunnel: w252 -> [w296]
            tunnel: w250 -> [w295]
            tunnel: [w294] -> w246
            tunnel: [w293] -> w245
            tunnel: w239 -> [w292]
            tunnel: [w292] -> w238
            tunnel: w234 -> [w291]
            tunnel: [w291] -> w233
            tunnel: w229 -> [w290]
            tunnel: [w290] -> w228
            tunnel: [w319] -> w247
            tunnel: w246 -> [w319]
            tunnel: w245 -> [w318]
            tunnel: [w317] -> w242
            tunnel: w238 -> [w316]
            tunnel: [w316] -> w237
            tunnel: w233 -> [w315]
            tunnel: [w315] -> w232
            tunnel: w228 -> [w314]
            tunnel: [w314] -> w227
            tunnel: [w329] -> w248
            tunnel: w247 -> [w329]
            tunnel: [w328] -> w243
            tunnel: w242 -> [w328]
            tunnel: w237 -> [w327]
            tunnel: w232 -> [w326]
            tunnel: w227 -> [w324]
            tunnel: [w327] -> w226
            tunnel: [w325] -> w225
            tunnel: [w324] -> w222
            tunnel: [w337] -> w249
            tunnel: w248 -> [w337]
            tunnel: [w336] -> w244
            tunnel: w243 -> [w336]
            tunnel: w226 -> [w334]
            tunnel: w225 -> [w335]
            tunnel: [w335] -> w224
            tunnel: [w333] -> w223
            tunnel: w222 -> [w332]
            tunnel: [w332] -> w221
            tunnel: [w345] -> _
            tunnel: w249 -> [w345]
            tunnel: [w344] -> _
            tunnel: w244 -> [w344]
            tunnel: w224 -> [w340]
            tunnel: w223 -> [w343]
            tunnel: [w343] -> _
            tunnel: w221 -> [w342]
            tunnel: [w341] -> _
            tunnel: [w340] -> _
            frame #0 {
              n79 = while {
                tunnel: w260 -> [w271]
                shift-right: [w275] -> w262
                shift-left: w261 -> [w276]
                tunnel: [w270] -> w259
                stop <- w264 stop-if-true
                w267 = -90.0 ("setpoint")
                # "Turns 90 dg right"
                n80 = call <vilib>:"ADI_IMU_ADIS16448_Get Angles.vi"("ADI IMU DevRef"=w271) -> ("IMU Angles Out"=w269:T17, "ADI IMU DevRef Out"=w270:T5)  [unwired: 7 in, 2 out]
                n81 = Unbundle By Name(w269) -> ("X Angle"=w268:dbl)
                n82 = Subtract(x=w268, y=w267) -> (x-y=w266:dbl)
                n83 = call-poly <vilib>:"PID.vi"("output range"=cluster{"output high":dbl, "output low":dbl} {"output high"=0.6, "output low"=-0.6}, "PID gains"=T15 {"proportional gain (Kc)"=-1.0, "integral time (Ti, min)"=0.0, "derivative time (Td, min)"=0.0}, "process variable"=w268, "setpoint"=w267) -> ("output"=w272:dbl)  [unwired: 6 in, 1 out]
                n84 = call-poly <vilib>:"WPI_RobotDriveArcadeDrive.vi"("Y axis value"=0.0 ("X axis value"), "X axis value"=w272, "RobotDriveDevRef"=w276) -> ("RobotDriveDevRef"=w278:T7)  [unwired: 1 in, 7 out]
                n85 = Absolute Value(x=w266) -> (abs(x)=w265:dbl)
                n86 = call <vilib>:"WPI_RobotDriveDelayAndUpdateSafety.vi"("Delay (s)"=0.1, "RobotDriveDevRef"=w278) -> ("RobotDriveDevRef 2"=w275:T7)  [unwired: 8 in, 1 out]
                n87 = Less?(x=w265, y=1.0) -> (x < y?=w264:bool)
              }
            }
            frame #1 {
              # "Drive for 1.5 seconds"
              n88 = call-poly <vilib>:"WPI_RobotDriveArcadeDrive.vi"("Y axis value"=-0.5 ("X axis value"), "X axis value"=0.0, "RobotDriveDevRef"=w284) -> ("RobotDriveDevRef"=w287:T7)  [unwired: 1 in, 7 out]
              n89 = call <vilib>:"WPI_RobotDriveDelayAndUpdateSafety.vi"("Delay (s)"=1.5, "RobotDriveDevRef"=w287) -> ("RobotDriveDevRef 2"=w283:T7)  [unwired: 8 in, 1 out]
            }
            frame #2 {
              n90 = while {
                shift-right: [w309] -> w293
                shift-left: w295 -> [w310]
                tunnel: [w304] -> w294
                tunnel: w296 -> [w305]
                stop <- w297 stop-if-true
                w298 = 0.0 ("setpoint")
                # "turns left 90dg"
                n91 = call <vilib>:"ADI_IMU_ADIS16448_Get Angles.vi"("ADI IMU DevRef"=w305) -> ("IMU Angles Out"=w303:T17, "ADI IMU DevRef Out"=w304:T5)  [unwired: 7 in, 2 out]
                n92 = Unbundle By Name(w303) -> ("X Angle"=w299:dbl)
                n93 = Subtract(x=w299, y=w298) -> (x-y=w302:dbl)
                n94 = call-poly <vilib>:"PID.vi"("output range"=cluster{"output high":dbl, "output low":dbl} {"output high"=0.6, "output low"=-0.6}, "PID gains"=T15 {"proportional gain (Kc)"=-1.0, "integral time (Ti, min)"=0.0, "derivative time (Td, min)"=0.0}, "process variable"=w299, "setpoint"=w298) -> ("output"=w306:dbl)  [unwired: 6 in, 1 out]
                n95 = call-poly <vilib>:"WPI_RobotDriveArcadeDrive.vi"("Y axis value"=0.0 ("X axis value"), "X axis value"=w306, "RobotDriveDevRef"=w310) -> ("RobotDriveDevRef"=w312:T7)  [unwired: 1 in, 7 out]
                n96 = Absolute Value(x=w302) -> (abs(x)=w301:dbl)
                n97 = call <vilib>:"WPI_RobotDriveDelayAndUpdateSafety.vi"("Delay (s)"=0.1, "RobotDriveDevRef"=w312) -> ("RobotDriveDevRef 2"=w309:T7)  [unwired: 8 in, 1 out]
                n98 = Less?(x=w301, y=1.0) -> (x < y?=w297:bool)
              }
            }
            frame #3 {
              # "drive forward for 1.5 \nseconds"
              n99 = call-poly <vilib>:"WPI_RobotDriveArcadeDrive.vi"("Y axis value"=-0.7 ("X axis value"), "X axis value"=0.0, "RobotDriveDevRef"=w318) -> ("RobotDriveDevRef"=w321:T7)  [unwired: 2 in, 6 out]
              n100 = call <vilib>:"WPI_RobotDriveDelayAndUpdateSafety.vi"("Delay (s)"=1.5, "RobotDriveDevRef"=w321) -> ("RobotDriveDevRef 2"=w317:T7)  [unwired: 8 in, 1 out]
            }
            frame #4 {
              w330 = T18 1 items=["PercentOutput"=0, "Position"=1, "Velocity"=2, "Current"=3, "Follower"=5, "MotionProfile"=6, "MotionMagic"=7, "MotionMagicArc"=8, "MotionProfileArc"=10, "Disabled"=15] ("Control Mode")
              n101 = call "CTRE_Phoenix_MotorControl_Set.vi"("Output"=29000.0, "Control Mode"=w330, "PhoenixMotorControlDevRef"=w326) -> ("PhoenixMotorControlDevRef"=w325:T8)  [unwired: 7 in, 1 out]
            }
            frame #5 {
              w338 = T18 1 items=["PercentOutput"=0, "Position"=1, "Velocity"=2, "Current"=3, "Follower"=5, "MotionProfile"=6, "MotionMagic"=7, "MotionMagicArc"=8, "MotionProfileArc"=10, "Disabled"=15] ("Control Mode")
              n102 = call "CTRE_Phoenix_MotorControl_Set.vi"("Output"=-8000.0, "Control Mode"=w338, "PhoenixMotorControlDevRef"=w334) -> ("PhoenixMotorControlDevRef"=w333:T8)  [unwired: 7 in, 1 out]
            }
            frame #6 {
              n103 = call-poly <vilib>:"WPI_SolenoidSet.vi"("Value"=WPI_SolenoidValue."Forward", "SolenoidDevRef"=w342) -> ("SolenoidDevRef"=w341:T13)  [unwired: 8 in, 1 out]
            }
          }
        }
      }
    }
    frame "4" {
      n104 = String Subset(string=w356, offset (0)=0, length (rest)=1 ("length (rest)")) -> (substring=w353:string)
      n105 = call-poly <vilib>:"WPI_SolenoidSet.vi"("Value"=WPI_SolenoidValue."Reverse", "SolenoidDevRef"=w348) -> ("SolenoidDevRef"=w347:T13)  [unwired: 8 in, 1 out]
      n106 = case shown="\"R\"" w353 {
        tunnel: w352 -> [w360 w405]
        tunnel: w351 -> [w371 _]
        tunnel: w350 -> [w370 _]
        tunnel: w347 -> [w372 _]
        frame "R" {
          n107 = flat-sequence {
            tunnel: w372 -> [w375]
            tunnel: w371 -> [w377]
            tunnel: w370 -> [w376]
            tunnel: [w376] -> w369
            tunnel: [w375] -> w368
            tunnel: [w374] -> w367
            tunnel: w360 -> [w373]
            tunnel: [w373] -> w358
            tunnel: w369 -> [w382]
            tunnel: w368 -> [w383]
            tunnel: w367 -> [w384]
            tunnel: [w384] -> w366
            tunnel: [w383] -> w364
            tunnel: [w381] -> w362
            tunnel: [w380] -> w359
            tunnel: w358 -> [w380]
            tunnel: w366 -> [w398]
            tunnel: [w398] -> w365
            tunnel: w364 -> [w397]
            tunnel: [w397] -> w363
            tunnel: w362 -> [w396]
            tunnel: [w396] -> w361
            tunnel: w359 -> [w389]
            tunnel: [w388] -> w357
            tunnel: w365 -> [w400]
            tunnel: w363 -> [w403]
            tunnel: w361 -> [w401]
            tunnel: [w402] -> _
            tunnel: [w401] -> _
            tunnel: [w400] -> _
            tunnel: w357 -> [w399]
            tunnel: [w399] -> _
            frame #0 {
              w378 = T18 1 items=["PercentOutput"=0, "Position"=1, "Velocity"=2, "Current"=3, "Follower"=5, "MotionProfile"=6, "MotionMagic"=7, "MotionMagicArc"=8, "MotionProfileArc"=10, "Disabled"=15] ("Control Mode")
              n108 = call "CTRE_Phoenix_MotorControl_Set.vi"("Output"=13000.0, "Control Mode"=w378, "PhoenixMotorControlDevRef"=w377) -> ("PhoenixMotorControlDevRef"=w374:T8)  [unwired: 7 in, 1 out]
            }
            frame #1 {
              w385 = T18 1 items=["PercentOutput"=0, "Position"=1, "Velocity"=2, "Current"=3, "Follower"=5, "MotionProfile"=6, "MotionMagic"=7, "MotionMagicArc"=8, "MotionProfileArc"=10, "Disabled"=15] ("Control Mode")
              n109 = call "CTRE_Phoenix_MotorControl_Set.vi"("Output"=-9200.0, "Control Mode"=w385, "PhoenixMotorControlDevRef"=w382) -> ("PhoenixMotorControlDevRef"=w381:T8)  [unwired: 7 in, 1 out]
            }
            frame #2 {
              # "stand still"
              # "turn for 1 second"
              n110 = call-poly <vilib>:"WPI_RobotDriveArcadeDrive.vi"("Y axis value"=-0.5 ("X axis value"), "X axis value"=0.0, "RobotDriveDevRef"=w389) -> ("RobotDriveDevRef"=w391:T7)  [unwired: 1 in, 7 out]
              n111 = call <vilib>:"WPI_RobotDriveDelayAndUpdateSafety.vi"("Delay (s)"=5.0, "RobotDriveDevRef"=w391) -> ("RobotDriveDevRef 2"=w390:T7)  [unwired: 8 in, 1 out]
              n112 = call-poly <vilib>:"WPI_RobotDriveArcadeDrive.vi"("Y axis value"=0.0 ("X axis value"), "X axis value"=0.0, "RobotDriveDevRef"=w390) -> ("RobotDriveDevRef"=w388:T7)  [unwired: 1 in, 7 out]
            }
            frame #3 {
              n113 = call-poly <vilib>:"WPI_SolenoidSet.vi"("Value"=WPI_SolenoidValue."Forward", "SolenoidDevRef"=w403) -> ("SolenoidDevRef"=w402:T13)  [unwired: 8 in, 1 out]
            }
          }
        }
        frame "L", Default {
          # "stand still"
          # "turn for 1 second"
          n114 = call-poly <vilib>:"WPI_RobotDriveArcadeDrive.vi"("Y axis value"=-0.5 ("X axis value"), "X axis value"=0.0, "RobotDriveDevRef"=w405) -> ("RobotDriveDevRef"=w408:T7)  [unwired: 1 in, 7 out]
          n115 = call <vilib>:"WPI_RobotDriveDelayAndUpdateSafety.vi"("Delay (s)"=4.0, "RobotDriveDevRef"=w408) -> ("RobotDriveDevRef 2"=w406:T7)  [unwired: 8 in, 1 out]
          n116 = call-poly <vilib>:"WPI_RobotDriveArcadeDrive.vi"("Y axis value"=0.0 ("X axis value"), "X axis value"=0.0, "RobotDriveDevRef"=w406) -> ()  [unwired: 1 in, 8 out]
        }
      }
    }
    frame "Practice 1" {
      # "stand still"
      # "turn for 1 second"
      n117 = call-poly <vilib>:"WPI_RobotDriveArcadeDrive.vi"("Y axis value"=-0.65 ("X axis value"), "X axis value"=0.0, "RobotDriveDevRef"=w413) -> ("RobotDriveDevRef"=w416:T7)  [unwired: 1 in, 7 out]
      n118 = call <vilib>:"WPI_RobotDriveDelayAndUpdateSafety.vi"("Delay (s)"=5.0, "RobotDriveDevRef"=w416) -> ("RobotDriveDevRef 2"=w414:T7)  [unwired: 8 in, 1 out]
      n119 = call-poly <vilib>:"WPI_RobotDriveArcadeDrive.vi"("Y axis value"=0.0 ("X axis value"), "X axis value"=0.0, "RobotDriveDevRef"=w414) -> ()  [unwired: 1 in, 8 out]
    }
    frame "5" {
      n120 = case shown="\"R\"" w424 {
        tunnel: w425 -> [w429 w467]
        tunnel: w422 -> [w427 _]
        tunnel: w421 -> [w428 _]
        tunnel: w423 -> [w426 _]
        frame "R" {
          n121 = flat-sequence {
            tunnel: w429 -> [w442]
            tunnel: w428 -> [w441]
            tunnel: w427 -> [w440]
            tunnel: [w441] -> w438
            tunnel: [w440] -> w437
            tunnel: w426 -> [w439]
            tunnel: [w439] -> w436
            tunnel: w438 -> [w453]
            tunnel: w437 -> [w452]
            tunnel: [w453] -> w435
            tunnel: [w451] -> w434
            tunnel: w436 -> [w450]
            tunnel: [w450] -> w433
            tunnel: w435 -> [w459]
            tunnel: w434 -> [w458]
            tunnel: [w458] -> w432
            tunnel: [w457] -> w431
            tunnel: w433 -> [w456]
            tunnel: [w456] -> w430
            tunnel: [w465] -> _
            tunnel: [w466] -> _
            tunnel: w432 -> [w466]
            tunnel: w431 -> [w465]
            tunnel: w430 -> [w464]
            tunnel: [w462] -> _
            frame #0 {
              # "stand still"
              # "turn for 1 second"
              n122 = call-poly <vilib>:"WPI_RobotDriveArcadeDrive.vi"("Y axis value"=-0.75 ("X axis value"), "X axis value"=0.0, "RobotDriveDevRef"=w442) -> ("RobotDriveDevRef"=w445:T7)  [unwired: 1 in, 7 out]
              n123 = call <vilib>:"WPI_RobotDriveDelayAndUpdateSafety.vi"("Delay (s)"=1.0, "RobotDriveDevRef"=w445) -> ("RobotDriveDevRef 2"=w443:T7)  [unwired: 8 in, 1 out]
              n124 = call-poly <vilib>:"WPI_RobotDriveArcadeDrive.vi"("Y axis value"=0.0 ("X axis value"), "X axis value"=0.0, "RobotDriveDevRef"=w443) -> ()  [unwired: 1 in, 8 out]
            }
            frame #1 {
              w454 = T18 1 items=["PercentOutput"=0, "Position"=1, "Velocity"=2, "Current"=3, "Follower"=5, "MotionProfile"=6, "MotionMagic"=7, "MotionMagicArc"=8, "MotionProfileArc"=10, "Disabled"=15] ("Control Mode")
              n125 = call "CTRE_Phoenix_MotorControl_Set.vi"("Output"=5000.0, "Control Mode"=w454, "PhoenixMotorControlDevRef"=w452) -> ("PhoenixMotorControlDevRef"=w451:T8)  [unwired: 7 in, 1 out]
            }
            frame #2 {
              w460 = T18 1 items=["PercentOutput"=0, "Position"=1, "Velocity"=2, "Current"=3, "Follower"=5, "MotionProfile"=6, "MotionMagic"=7, "MotionMagicArc"=8, "MotionProfileArc"=10, "Disabled"=15] ("Control Mode")
              n126 = call "CTRE_Phoenix_MotorControl_Set.vi"("Output"=8000.0, "Control Mode"=w460, "PhoenixMotorControlDevRef"=w459) -> ("PhoenixMotorControlDevRef"=w457:T8)  [unwired: 7 in, 1 out]
            }
            frame #3 {
              n127 = call-poly <vilib>:"WPI_SolenoidSet.vi"("Value"=WPI_SolenoidValue."Forward", "SolenoidDevRef"=w464) -> ("SolenoidDevRef"=w462:T13)  [unwired: 8 in, 1 out]
            }
          }
        }
        frame "L", Default {
          # "stand still"
          # "turn for 1 second"
          n128 = call-poly <vilib>:"WPI_RobotDriveArcadeDrive.vi"("Y axis value"=-0.75 ("X axis value"), "X axis value"=0.0, "RobotDriveDevRef"=w467) -> ("RobotDriveDevRef"=w470:T7)  [unwired: 1 in, 7 out]
          n129 = call <vilib>:"WPI_RobotDriveDelayAndUpdateSafety.vi"("Delay (s)"=0.5, "RobotDriveDevRef"=w470) -> ("RobotDriveDevRef 2"=w468:T7)  [unwired: 8 in, 1 out]
          n130 = call-poly <vilib>:"WPI_RobotDriveArcadeDrive.vi"("Y axis value"=0.0 ("X axis value"), "X axis value"=0.0, "RobotDriveDevRef"=w468) -> ()  [unwired: 1 in, 8 out]
        }
      }
    }
    frame "3" {
      # "turn for 1 second"
      # "turn for 1 second"
      # "Drive for 1.5 seconds"
      # "turn for 1 second"
      # "stand still"
      # "turn for 1 second"
      n131 = call-poly <vilib>:"WPI_RobotDriveArcadeDrive.vi"("Y axis value"=-1.0 ("X axis value"), "X axis value"=0.0, "RobotDriveDevRef"=w475) -> ("RobotDriveDevRef"=w493:T7)  [unwired: 1 in, 7 out]
      n132 = call <vilib>:"WPI_RobotDriveDelayAndUpdateSafety.vi"("Delay (s)"=0.1, "RobotDriveDevRef"=w493) -> ("RobotDriveDevRef 2"=w494:T7)  [unwired: 8 in, 1 out]
      n133 = call-poly <vilib>:"WPI_RobotDriveArcadeDrive.vi"("Y axis value"=0.0 ("X axis value"), "X axis value"=0.0, "RobotDriveDevRef"=w494) -> ("RobotDriveDevRef"=w496:T7)  [unwired: 1 in, 7 out]
      n134 = call-poly <vilib>:"WPI_RobotDriveArcadeDrive.vi"("Y axis value"=0.0 ("X axis value"), "X axis value"=0.0, "RobotDriveDevRef"=w496) -> ("RobotDriveDevRef"=w495:T7)  [unwired: 1 in, 7 out]
      n135 = call <vilib>:"WPI_RobotDriveDelayAndUpdateSafety.vi"("Delay (s)"=0.1, "RobotDriveDevRef"=w495) -> ("RobotDriveDevRef 2"=w498:T7)  [unwired: 8 in, 1 out]
      n136 = call-poly <vilib>:"WPI_RobotDriveArcadeDrive.vi"("Y axis value"=-1.0 ("X axis value"), "X axis value"=0.0, "RobotDriveDevRef"=w498) -> ("RobotDriveDevRef"=w497:T7)  [unwired: 1 in, 7 out]
      n137 = call <vilib>:"WPI_RobotDriveDelayAndUpdateSafety.vi"("Delay (s)"=1.5, "RobotDriveDevRef"=w497) -> ("RobotDriveDevRef 2"=w500:T7)  [unwired: 8 in, 1 out]
      n138 = call-poly <vilib>:"WPI_RobotDriveArcadeDrive.vi"("Y axis value"=-1.0 ("X axis value"), "X axis value"=0.0, "RobotDriveDevRef"=w500) -> ("RobotDriveDevRef"=w499:T7)  [unwired: 1 in, 7 out]
      n139 = call <vilib>:"WPI_RobotDriveDelayAndUpdateSafety.vi"("Delay (s)"=0.1, "RobotDriveDevRef"=w499) -> ("RobotDriveDevRef 2"=w502:T7)  [unwired: 8 in, 1 out]
      n140 = call-poly <vilib>:"WPI_RobotDriveArcadeDrive.vi"("Y axis value"=-1.0 ("X axis value"), "X axis value"=0.0, "RobotDriveDevRef"=w502) -> ("RobotDriveDevRef"=w501:T7)  [unwired: 2 in, 6 out]
      n141 = call <vilib>:"WPI_RobotDriveDelayAndUpdateSafety.vi"("Delay (s)"=0.5, "RobotDriveDevRef"=w501) -> ()  [unwired: 8 in, 2 out]
    }
    frame "6" {
      n142 = String Subset(string=w504, offset (0)=0, length (rest)=1 ("length (rest)")) -> (substring=w503:string)
      n143 = case shown="\"True\"" w503 {
        tunnel: w511 -> [w513 w526]
        tunnel: w510 -> [_ w525]
        tunnel: w509 -> [_ w524]
        tunnel: w508 -> [_ w523]
        tunnel: w507 -> [_ w521]
        frame "False", Default {
          # "stand still"
          # "turn for 1 second"
          n144 = call-poly <vilib>:"WPI_RobotDriveArcadeDrive.vi"("Y axis value"=-0.5 ("X axis value"), "X axis value"=0.0, "RobotDriveDevRef"=w513) -> ("RobotDriveDevRef"=w516:T7)  [unwired: 1 in, 7 out]
          n145 = call <vilib>:"WPI_RobotDriveDelayAndUpdateSafety.vi"("Delay (s)"=5.0, "RobotDriveDevRef"=w516) -> ("RobotDriveDevRef 2"=w514:T7)  [unwired: 8 in, 1 out]
          n146 = call-poly <vilib>:"WPI_RobotDriveArcadeDrive.vi"("Y axis value"=0.0 ("X axis value"), "X axis value"=0.0, "RobotDriveDevRef"=w514) -> ()  [unwired: 1 in, 8 out]
        }
        frame "True" {
          # "stand still"
          # "turn for 1 second"
          n147 = call-poly <vilib>:"WPI_SolenoidSet.vi"("Value"=WPI_SolenoidValue."Reverse", "SolenoidDevRef"=w521) -> ("SolenoidDevRef"=w520:T13)  [unwired: 8 in, 1 out]
          n148 = call-poly <vilib>:"WPI_RobotDriveArcadeDrive.vi"("Y axis value"=-0.5 ("X axis value"), "X axis value"=0.0, "RobotDriveDevRef"=w526) -> ("RobotDriveDevRef"=w530:T7)  [unwired: 1 in, 7 out]
          n149 = call <vilib>:"WPI_RobotDriveDelayAndUpdateSafety.vi"("Delay (s)"=5.0, "RobotDriveDevRef"=w530) -> ("RobotDriveDevRef 2"=w528:T7)  [unwired: 8 in, 1 out]
          n150 = call-poly <vilib>:"WPI_RobotDriveArcadeDrive.vi"("Y axis value"=0.0 ("X axis value"), "X axis value"=0.0, "RobotDriveDevRef"=w528) -> ("RobotDriveDevRef"=w527:T7)  [unwired: 1 in, 7 out]
          n151 = flat-sequence {
            tunnel: w520 -> [w558]
            tunnel: w525 -> [w560]
            tunnel: w524 -> [w559]
            tunnel: [w559] -> w554
            tunnel: [w558] -> w553
            tunnel: [w557] -> w552
            tunnel: w527 -> [w556]
            tunnel: [w556] -> w551
            tunnel: w523 -> [w555]
            tunnel: [w555] -> w550
            tunnel: w554 -> [w566]
            tunnel: w553 -> [w567]
            tunnel: w552 -> [w568]
            tunnel: [w568] -> w549
            tunnel: [w567] -> w548
            tunnel: [w565] -> w547
            tunnel: [w564] -> w546
            tunnel: w551 -> [w564]
            tunnel: [w563] -> w545
            tunnel: w550 -> [w563]
            tunnel: w549 -> [w576]
            tunnel: [w576] -> w544
            tunnel: w548 -> [w575]
            tunnel: [w575] -> w543
            tunnel: w547 -> [w577]
            tunnel: [w577] -> w542
            tunnel: w546 -> [w574]
            tunnel: [w573] -> w541
            tunnel: w545 -> [w572]
            tunnel: [w571] -> w540
            tunnel: w544 -> [w607]
            tunnel: [w607] -> w539
            tunnel: w543 -> [w606]
            tunnel: [w606] -> w538
            tunnel: w542 -> [w605]
            tunnel: [w605] -> w537
            tunnel: w541 -> [w597]
            tunnel: [w596] -> w536
            tunnel: [w595] -> w535
            tunnel: w540 -> [w595]
            tunnel: w539 -> [w610]
            tunnel: w538 -> [w613]
            tunnel: w537 -> [w611]
            tunnel: [w612] -> _
            tunnel: [w611] -> _
            tunnel: [w610] -> _
            tunnel: [w609] -> _
            tunnel: w536 -> [w609]
            tunnel: [w608] -> _
            tunnel: w535 -> [w608]
            frame #0 {
              w561 = T18 1 items=["PercentOutput"=0, "Position"=1, "Velocity"=2, "Current"=3, "Follower"=5, "MotionProfile"=6, "MotionMagic"=7, "MotionMagicArc"=8, "MotionProfileArc"=10, "Disabled"=15] ("Control Mode")
              n152 = call "CTRE_Phoenix_MotorControl_Set.vi"("Output"=5000.0, "Control Mode"=w561, "PhoenixMotorControlDevRef"=w560) -> ("PhoenixMotorControlDevRef"=w557:T8)  [unwired: 7 in, 1 out]
            }
            frame #1 {
              w569 = T18 1 items=["PercentOutput"=0, "Position"=1, "Velocity"=2, "Current"=3, "Follower"=5, "MotionProfile"=6, "MotionMagic"=7, "MotionMagicArc"=8, "MotionProfileArc"=10, "Disabled"=15] ("Control Mode")
              n153 = call "CTRE_Phoenix_MotorControl_Set.vi"("Output"=8000.0, "Control Mode"=w569, "PhoenixMotorControlDevRef"=w566) -> ("PhoenixMotorControlDevRef"=w565:T8)  [unwired: 7 in, 1 out]
            }
            frame #2 {
              n154 = while {
                tunnel: w572 -> [w586]
                shift-right: [w590] -> w573
                shift-left: w574 -> [w591]
                tunnel: [w585] -> w571
                stop <- w579 stop-if-true
                w582 = -90.0 ("setpoint")
                # "turn for 1 second"
                n155 = call <vilib>:"ADI_IMU_ADIS16448_Get Angles.vi"("ADI IMU DevRef"=w586) -> ("IMU Angles Out"=w584:T17, "ADI IMU DevRef Out"=w585:T5)  [unwired: 7 in, 2 out]
                n156 = Unbundle By Name(w584) -> ("X Angle"=w583:dbl)
                n157 = Subtract(x=w583, y=w582) -> (x-y=w581:dbl)
                n158 = call-poly <vilib>:"PID.vi"("output range"=cluster{"output high":dbl, "output low":dbl} {"output high"=0.6, "output low"=-0.6}, "PID gains"=T15 {"proportional gain (Kc)"=-1.0, "integral time (Ti, min)"=0.0, "derivative time (Td, min)"=0.0}, "process variable"=w583, "setpoint"=w582) -> ("output"=w587:dbl)  [unwired: 6 in, 1 out]
                n159 = call-poly <vilib>:"WPI_RobotDriveArcadeDrive.vi"("Y axis value"=0.0 ("X axis value"), "X axis value"=w587, "RobotDriveDevRef"=w591) -> ("RobotDriveDevRef"=w593:T7)  [unwired: 1 in, 7 out]
                n160 = Absolute Value(x=w581) -> (abs(x)=w580:dbl)
                n161 = call <vilib>:"WPI_RobotDriveDelayAndUpdateSafety.vi"("Delay (s)"=0.1, "RobotDriveDevRef"=w593) -> ("RobotDriveDevRef 2"=w590:T7)  [unwired: 8 in, 1 out]
                n162 = Less?(x=w580, y=1.0) -> (x < y?=w579:bool)
              }
            }
            frame #3 {
              # "stand still"
              # "turn for 1 second"
              n163 = call-poly <vilib>:"WPI_RobotDriveArcadeDrive.vi"("Y axis value"=-0.5 ("X axis value"), "X axis value"=0.0, "RobotDriveDevRef"=w597) -> ("RobotDriveDevRef"=w600:T7)  [unwired: 1 in, 7 out]
              n164 = call <vilib>:"WPI_RobotDriveDelayAndUpdateSafety.vi"("Delay (s)"=2.0, "RobotDriveDevRef"=w600) -> ("RobotDriveDevRef 2"=w598:T7)  [unwired: 8 in, 1 out]
              n165 = call-poly <vilib>:"WPI_RobotDriveArcadeDrive.vi"("Y axis value"=0.0 ("X axis value"), "X axis value"=0.0, "RobotDriveDevRef"=w598) -> ("RobotDriveDevRef"=w596:T7)  [unwired: 1 in, 7 out]
            }
            frame #4 {
              n166 = call-poly <vilib>:"WPI_SolenoidSet.vi"("Value"=WPI_SolenoidValue."Forward", "SolenoidDevRef"=w613) -> ("SolenoidDevRef"=w612:T13)  [unwired: 8 in, 1 out]
            }
          }
        }
      }
    }
    frame "8" {
      n167 = String Subset(string=w615, offset (0)=0, length (rest)=1 ("length (rest)")) -> (substring=w625:string)
      n168 = call-poly <vilib>:"WPI_SolenoidSet.vi"("Value"=WPI_SolenoidValue."Reverse", "SolenoidDevRef"=w616) -> ("SolenoidDevRef"=w621:T13)  [unwired: 8 in, 1 out]
      n169 = case shown="\"L\"" w625 {
        tunnel: w619 -> [_ w648]
        tunnel: w618 -> [_ w647]
        tunnel: w621 -> [_ w646]
        tunnel: w620 -> [_ w645]
        tunnel: w617 -> [w626 w644]
        frame "R", Default {
          # "stand still"
          # "Drive Straight to \nBaseline"
          n170 = call-poly <vilib>:"WPI_RobotDriveArcadeDrive.vi"("Y axis value"=-0.5 ("X axis value"), "X axis value"=0.0, "RobotDriveDevRef"=w626) -> ("RobotDriveDevRef"=w629:T7)  [unwired: 1 in, 7 out]
          n171 = call <vilib>:"WPI_RobotDriveDelayAndUpdateSafety.vi"("Delay (s)"=5.0, "RobotDriveDevRef"=w629) -> ("RobotDriveDevRef 2"=w627:T7)  [unwired: 8 in, 1 out]
          n172 = call-poly <vilib>:"WPI_RobotDriveArcadeDrive.vi"("Y axis value"=0.0 ("X axis value"), "X axis value"=0.0, "RobotDriveDevRef"=w627) -> ()  [unwired: 1 in, 8 out]
        }
        frame "L" {
          n173 = flat-sequence {
            tunnel: w648 -> [w668]
            tunnel: w647 -> [w665]
            tunnel: w646 -> [w669]
            tunnel: w645 -> [w670]
            tunnel: w644 -> [w671]
            tunnel: [w671] -> w643
            tunnel: [w670] -> w641
            tunnel: [w669] -> w639
            tunnel: [w664] -> w637
            tunnel: [w668] -> w635
            tunnel: w643 -> [w679]
            tunnel: [w679] -> w642
            tunnel: w641 -> [w678]
            tunnel: [w678] -> w640
            tunnel: w639 -> [w677]
            tunnel: [w677] -> w638
            tunnel: w637 -> [w676]
            tunnel: [w676] -> w636
            tunnel: w635 -> [w673]
            tunnel: [w672] -> w634
            tunnel: [w687] -> w663
            tunnel: [w683] -> w662
            tunnel: [w682] -> w661
            tunnel: [w681] -> w660
            tunnel: [w680] -> w659
            tunnel: w642 -> [w689]
            tunnel: w640 -> [w683]
            tunnel: w638 -> [w682]
            tunnel: w636 -> [w681]
            tunnel: w634 -> [w680]
            tunnel: w663 -> [w693]
            tunnel: w662 -> [w692]
            tunnel: w661 -> [w696]
            tunnel: [w696] -> w658
            tunnel: w660 -> [w695]
            tunnel: [w695] -> w657
            tunnel: w659 -> [w694]
            tunnel: [w694] -> w656
            tunnel: [w691] -> w655
            tunnel: [w690] -> w654
            tunnel: [w726] -> w653
            tunnel: [w715] -> w652
            tunnel: [w714] -> w651
            tunnel: [w725] -> w650
            tunnel: [w724] -> w649
            tunnel: w654 -> [w724]
            tunnel: w655 -> [w716]
            tunnel: w656 -> [w714]
            tunnel: w657 -> [w715]
            tunnel: w658 -> [w726]
            tunnel: w653 -> [w730]
            tunnel: w652 -> [w733]
            tunnel: [w733] -> _
            tunnel: w651 -> [w732]
            tunnel: [w732] -> _
            tunnel: [w729] -> _
            tunnel: [w728] -> _
            tunnel: w650 -> [w728]
            tunnel: [w727] -> _
            tunnel: w649 -> [w727]
            frame #0 {
              w666 = T18 1 items=["PercentOutput"=0, "Position"=1, "Velocity"=2, "Current"=3, "Follower"=5, "MotionProfile"=6, "MotionMagic"=7, "MotionMagicArc"=8, "MotionProfileArc"=10, "Disabled"=15] ("Control Mode")
              n174 = call "CTRE_Phoenix_MotorControl_Set.vi"("Output"=13000.0, "Control Mode"=w666, "PhoenixMotorControlDevRef"=w665) -> ("PhoenixMotorControlDevRef"=w664:T8)  [unwired: 7 in, 1 out]
            }
            frame #1 {
              w674 = T18 1 items=["PercentOutput"=0, "Position"=1, "Velocity"=2, "Current"=3, "Follower"=5, "MotionProfile"=6, "MotionMagic"=7, "MotionMagicArc"=8, "MotionProfileArc"=10, "Disabled"=15] ("Control Mode")
              n175 = call "CTRE_Phoenix_MotorControl_Set.vi"("Output"=-9200.0, "Control Mode"=w674, "PhoenixMotorControlDevRef"=w673) -> ("PhoenixMotorControlDevRef"=w672:T8)  [unwired: 7 in, 1 out]
            }
            frame #2 {
              n176 = call-poly <vilib>:"WPI_RobotDriveArcadeDrive.vi"("Y axis value"=-0.5, "X axis value"=0.0, "RobotDriveDevRef"=w689) -> ("RobotDriveDevRef"=w688:T7)  [unwired: 6 in, 2 out]
              n177 = call <vilib>:"WPI_RobotDriveDelayAndUpdateSafety.vi"("Delay (s)"=5.5, "RobotDriveDevRef"=w688) -> ("RobotDriveDevRef 2"=w687:T7)  [unwired: 8 in, 1 out]
            }
            frame #3 {
              n178 = while {
                tunnel: w692 -> [w705]
                shift-right: [w709] -> w691
                shift-left: w693 -> [w710]
                tunnel: [w704] -> w690
                stop <- w698 stop-if-true
                w701 = -90.0 ("setpoint")
                # "Turns 90 dg right"
                n179 = call <vilib>:"ADI_IMU_ADIS16448_Get Angles.vi"("ADI IMU DevRef"=w705) -> ("IMU Angles Out"=w703:T17, "ADI IMU DevRef Out"=w704:T5)  [unwired: 7 in, 2 out]
                n180 = Unbundle By Name(w703) -> ("X Angle"=w702:dbl)
                n181 = Subtract(x=w702, y=w701) -> (x-y=w700:dbl)
                n182 = call-poly <vilib>:"PID.vi"("output range"=cluster{"output high":dbl, "output low":dbl} {"output high"=0.5, "output low"=-0.5}, "PID gains"=T15 {"proportional gain (Kc)"=0.1, "integral time (Ti, min)"=0.0, "derivative time (Td, min)"=0.0}, "process variable"=w702, "setpoint"=w701) -> ("output"=w706:dbl)  [unwired: 6 in, 1 out]
                n183 = call-poly <vilib>:"WPI_RobotDriveArcadeDrive.vi"("Y axis value"=0.0 ("X axis value"), "X axis value"=w706, "RobotDriveDevRef"=w710) -> ("RobotDriveDevRef"=w712:T7)  [unwired: 1 in, 7 out]
                n184 = Absolute Value(x=w700) -> (abs(x)=w699:dbl)
                n185 = call <vilib>:"WPI_RobotDriveDelayAndUpdateSafety.vi"("Delay (s)"=0.1, "RobotDriveDevRef"=w712) -> ("RobotDriveDevRef 2"=w709:T7)  [unwired: 8 in, 1 out]
                n186 = Less?(x=w699, y=1.0) -> (x < y?=w698:bool)
              }
            }
            frame #4 {
              n187 = call-poly <vilib>:"WPI_RobotDriveArcadeDrive.vi"("Y axis value"=-0.5, "X axis value"=0.0, "RobotDriveDevRef"=w716) -> ("RobotDriveDevRef"=w723:T7)  [unwired: 6 in, 2 out]
              n188 = call <vilib>:"WPI_RobotDriveDelayAndUpdateSafety.vi"("Delay (s)"=2.0, "RobotDriveDevRef"=w723) -> ("RobotDriveDevRef 2"=w719:T7)  [unwired: 8 in, 1 out]
              n189 = call-poly <vilib>:"WPI_RobotDriveArcadeDrive.vi"("Y axis value"=0.0, "X axis value"=0.0, "RobotDriveDevRef"=w719) -> ("RobotDriveDevRef"=w725:T7)  [unwired: 6 in, 2 out]
            }
            frame #5 {
              n190 = call-poly <vilib>:"WPI_SolenoidSet.vi"("Value"=WPI_SolenoidValue."Forward", "SolenoidDevRef"=w730) -> ("SolenoidDevRef"=w729:T13)  [unwired: 8 in, 1 out]
            }
          }
        }
      }
    }
    frame "9" {
      n191 = String Subset(string=w740, offset (0)=0, length (rest)=1 ("length (rest)")) -> (substring=w739:string)
      n192 = call-poly <vilib>:"WPI_SolenoidSet.vi"("Value"=WPI_SolenoidValue."Reverse", "SolenoidDevRef"=w735) -> ("SolenoidDevRef"=w734:T13)  [unwired: 8 in, 1 out]
      n193 = case shown="\"R\"" w739 {
        tunnel: w744 -> [_ w767]
        tunnel: w743 -> [_ w766]
        tunnel: w734 -> [_ w765]
        tunnel: w742 -> [_ w764]
        tunnel: w741 -> [w745 w763]
        frame "L", Default {
          # "stand still"
          # "Drive Straight to \nBaseline"
          n194 = call-poly <vilib>:"WPI_RobotDriveArcadeDrive.vi"("Y axis value"=-0.5 ("X axis value"), "X axis value"=0.0, "RobotDriveDevRef"=w745) -> ("RobotDriveDevRef"=w748:T7)  [unwired: 1 in, 7 out]
          n195 = call <vilib>:"WPI_RobotDriveDelayAndUpdateSafety.vi"("Delay (s)"=5.0, "RobotDriveDevRef"=w748) -> ("RobotDriveDevRef 2"=w746:T7)  [unwired: 8 in, 1 out]
          n196 = call-poly <vilib>:"WPI_RobotDriveArcadeDrive.vi"("Y axis value"=0.0 ("X axis value"), "X axis value"=0.0, "RobotDriveDevRef"=w746) -> ()  [unwired: 1 in, 8 out]
        }
        frame "R" {
          n197 = flat-sequence {
            tunnel: w767 -> [w787]
            tunnel: w766 -> [w784]
            tunnel: w765 -> [w788]
            tunnel: w764 -> [w789]
            tunnel: w763 -> [w790]
            tunnel: [w790] -> w762
            tunnel: [w789] -> w760
            tunnel: [w788] -> w758
            tunnel: [w783] -> w756
            tunnel: [w787] -> w754
            tunnel: w762 -> [w798]
            tunnel: [w798] -> w761
            tunnel: w760 -> [w797]
            tunnel: [w797] -> w759
            tunnel: w758 -> [w796]
            tunnel: [w796] -> w757
            tunnel: w756 -> [w795]
            tunnel: [w795] -> w755
            tunnel: w754 -> [w792]
            tunnel: [w791] -> w753
            tunnel: [w806] -> w782
            tunnel: [w802] -> w781
            tunnel: [w801] -> w780
            tunnel: [w800] -> w779
            tunnel: [w799] -> w778
            tunnel: w761 -> [w808]
            tunnel: w759 -> [w802]
            tunnel: w757 -> [w801]
            tunnel: w755 -> [w800]
            tunnel: w753 -> [w799]
            tunnel: w782 -> [w812]
            tunnel: w781 -> [w811]
            tunnel: w780 -> [w815]
            tunnel: [w815] -> w777
            tunnel: w779 -> [w814]
            tunnel: [w814] -> w776
            tunnel: w778 -> [w813]
            tunnel: [w813] -> w775
            tunnel: [w810] -> w774
            tunnel: [w809] -> w773
            tunnel: [w845] -> w772
            tunnel: [w834] -> w771
            tunnel: [w833] -> w770
            tunnel: [w844] -> w769
            tunnel: [w843] -> w768
            tunnel: w773 -> [w843]
            tunnel: w774 -> [w835]
            tunnel: w775 -> [w833]
            tunnel: w776 -> [w834]
            tunnel: w777 -> [w845]
            tunnel: w772 -> [w849]
            tunnel: w771 -> [w852]
            tunnel: [w852] -> _
            tunnel: w770 -> [w851]
            tunnel: [w851] -> _
            tunnel: [w848] -> _
            tunnel: [w847] -> _
            tunnel: w769 -> [w847]
            tunnel: [w846] -> _
            tunnel: w768 -> [w846]
            frame #0 {
              w785 = T18 1 items=["PercentOutput"=0, "Position"=1, "Velocity"=2, "Current"=3, "Follower"=5, "MotionProfile"=6, "MotionMagic"=7, "MotionMagicArc"=8, "MotionProfileArc"=10, "Disabled"=15] ("Control Mode")
              n198 = call "CTRE_Phoenix_MotorControl_Set.vi"("Output"=13000.0, "Control Mode"=w785, "PhoenixMotorControlDevRef"=w784) -> ("PhoenixMotorControlDevRef"=w783:T8)  [unwired: 7 in, 1 out]
            }
            frame #1 {
              w793 = T18 1 items=["PercentOutput"=0, "Position"=1, "Velocity"=2, "Current"=3, "Follower"=5, "MotionProfile"=6, "MotionMagic"=7, "MotionMagicArc"=8, "MotionProfileArc"=10, "Disabled"=15] ("Control Mode")
              n199 = call "CTRE_Phoenix_MotorControl_Set.vi"("Output"=-9200.0, "Control Mode"=w793, "PhoenixMotorControlDevRef"=w792) -> ("PhoenixMotorControlDevRef"=w791:T8)  [unwired: 7 in, 1 out]
            }
            frame #2 {
              n200 = call-poly <vilib>:"WPI_RobotDriveArcadeDrive.vi"("Y axis value"=-0.5, "X axis value"=0.0, "RobotDriveDevRef"=w808) -> ("RobotDriveDevRef"=w807:T7)  [unwired: 6 in, 2 out]
              n201 = call <vilib>:"WPI_RobotDriveDelayAndUpdateSafety.vi"("Delay (s)"=5.5, "RobotDriveDevRef"=w807) -> ("RobotDriveDevRef 2"=w806:T7)  [unwired: 8 in, 1 out]
            }
            frame #3 {
              n202 = while {
                tunnel: w811 -> [w824]
                shift-right: [w828] -> w810
                shift-left: w812 -> [w829]
                tunnel: [w823] -> w809
                stop <- w817 stop-if-true
                w820 = 90.0 ("setpoint")
                # "Turns 90 dg right"
                n203 = call <vilib>:"ADI_IMU_ADIS16448_Get Angles.vi"("ADI IMU DevRef"=w824) -> ("IMU Angles Out"=w822:T17, "ADI IMU DevRef Out"=w823:T5)  [unwired: 7 in, 2 out]
                n204 = Unbundle By Name(w822) -> ("X Angle"=w821:dbl)
                n205 = Subtract(x=w821, y=w820) -> (x-y=w819:dbl)
                n206 = call-poly <vilib>:"PID.vi"("output range"=cluster{"output high":dbl, "output low":dbl} {"output high"=0.5, "output low"=-0.5}, "PID gains"=T15 {"proportional gain (Kc)"=-0.1, "integral time (Ti, min)"=0.0, "derivative time (Td, min)"=0.0}, "process variable"=w821, "setpoint"=w820) -> ("output"=w825:dbl)  [unwired: 6 in, 1 out]
                n207 = call-poly <vilib>:"WPI_RobotDriveArcadeDrive.vi"("Y axis value"=0.0 ("X axis value"), "X axis value"=w825, "RobotDriveDevRef"=w829) -> ("RobotDriveDevRef"=w831:T7)  [unwired: 1 in, 7 out]
                n208 = Absolute Value(x=w819) -> (abs(x)=w818:dbl)
                n209 = call <vilib>:"WPI_RobotDriveDelayAndUpdateSafety.vi"("Delay (s)"=0.1, "RobotDriveDevRef"=w831) -> ("RobotDriveDevRef 2"=w828:T7)  [unwired: 8 in, 1 out]
                n210 = Less?(x=w818, y=1.0) -> (x < y?=w817:bool)
              }
            }
            frame #4 {
              n211 = call-poly <vilib>:"WPI_RobotDriveArcadeDrive.vi"("Y axis value"=-0.5, "X axis value"=0.0, "RobotDriveDevRef"=w835) -> ("RobotDriveDevRef"=w842:T7)  [unwired: 6 in, 2 out]
              n212 = call <vilib>:"WPI_RobotDriveDelayAndUpdateSafety.vi"("Delay (s)"=2.0, "RobotDriveDevRef"=w842) -> ("RobotDriveDevRef 2"=w838:T7)  [unwired: 8 in, 1 out]
              n213 = call-poly <vilib>:"WPI_RobotDriveArcadeDrive.vi"("Y axis value"=0.0, "X axis value"=0.0, "RobotDriveDevRef"=w838) -> ("RobotDriveDevRef"=w844:T7)  [unwired: 6 in, 2 out]
            }
            frame #5 {
              n214 = call-poly <vilib>:"WPI_SolenoidSet.vi"("Value"=WPI_SolenoidValue."Forward", "SolenoidDevRef"=w849) -> ("SolenoidDevRef"=w848:T13)  [unwired: 8 in, 1 out]
            }
          }
        }
      }
    }
  }
